vi "GUI.vi"() -> ()   [LabVIEW 2021]
uses:
  <vilib>/Utility/sysdir.llb/System Directory Type.ctl
  Jumps_Globals.vi
  Stevci_Globals.vi
  belezenje.vi
  filePath.vi
  senzorji.vi
  Jump_Globals.vi
  <vilib>/express/express arith-compare/Formula/XNode/ExpressFormulaBlockNode.xnode
panel:
  out "date/time string":string
  out "Time Stamp":timestamp
  out "Start time":string
  in  "?":bool
  out "error out 6":errorcluster
  out "error out 5":errorcluster
  out "error out 4":errorcluster
  out "error out 3":errorcluster
  out "error out 2":errorcluster
  out "error out":errorcluster
  in  "Writing":string[](array[string])
  in  "ID_prejsnji_set6":dbl
  in  "ID_prejsnji_set5":dbl
  in  "ID_prejsnji_set4":dbl
  in  "ID_prejsnji_set3":dbl
  in  "ID_prejsnji_set2":dbl
  in  "ID_prejsnji_set1":dbl
  in  "?":bool
  in  "Lokalni Stevec 6":dbl
  in  "Lokalni Stevec 5":dbl
  in  "Lokalni Stevec 4":dbl
  in  "Lokalni Stevec 3":dbl
  in  "Lokalni Stevec 2":dbl
  in  "?":bool
  in  "Lokalni Stevec":dbl
  in  "?":enum32{"Senzorji", "Tekma", "Set", "Tocka"}(tab)
  out "baterija 6":dbl
  out "baterija 5":dbl
  out "baterija 4":dbl
  out "baterija 3":dbl
  out "baterija 2":dbl
  out "baterija 1":dbl
  out "Senzor 6":bool
  out "Senzor 5":bool
  out "Senzor 4":bool
  out "Senzor 3":bool
  out "Senzor 2":bool
  out "Senzor 1":bool
  out "Stevilo skokov tekma":dbl
  out "Povprecje2_tekma":dbl
  in  "String":string
  out "igralec1":string
  out "igralec2":string
  out "igralec3":string
  out "igralec4":string
  out "igralec5":string
  out "igralec6":string
  in  "String 2":string
  in  "String 3":string
  in  "String 4":string
  in  "String 5":string
  in  "String 6":string
  out "Povprecje1_tekma":dbl
  out "Povprecje3_tekma":dbl
  out "Povprecje4_tekma":dbl
  out "Povprecje5_tekma":dbl
  out "Povprecje6_tekma":dbl
  out "Stevilo skokov tekma 2":dbl
  out "Stevilo skokov tekma 3":dbl
  out "Stevilo skokov tekma 4":dbl
  out "Stevilo skokov tekma 5":dbl
  out "Stevilo skokov tekma 6":dbl
  out "Povprecje2_set":dbl
  out "igralec1 3":string
  out "igralec2 3":string
  out "igralec3 3":string
  out "igralec4 3":string
  out "igralec5 3":string
  out "igralec6 3":string
  in  "String 7":string
  in  "String 18":string
  in  "String 13":string
  in  "String 14":string
  in  "String 11":string
  in  "String 10":string
  out "Povprecje1_set":dbl
  out "Povprecje3_set":dbl
  out "Povprecje4_set":dbl
  out "Povprecje5_set":dbl
  out "Povprecje6_set":dbl
  out "Stevilo skokov set":dbl
  out "Stevilo skokov set 2":dbl
  out "Stevilo skokov set 3":dbl
  out "Stevilo skokov set 4":dbl
  out "Stevilo skokov set 5":dbl
  out "Stevilo skokov set 6":dbl
  out "Povprecje2_tocka":dbl
  out "igralec1 2":string
  out "igralec2 2":string
  out "igralec3 2":string
  out "igralec4 2":string
  out "igralec5 2":string
  out "igralec6 2":string
  in  "String 17":string
  in  "String 16":string
  in  "String 8":string
  in  "String 9":string
  in  "String 15":string
  in  "String 12":string
  out "Povprecje1_tocka":dbl
  out "Povprecje3_tocka":dbl
  out "Povprecje4_tocka":dbl
  out "Povprecje5_tocka":dbl
  out "Povprecje6_tocka":dbl
  out "Stevilo skokov tocka":dbl
  out "Stevilo skokov tocka 2":dbl
  out "Stevilo skokov tocka 3":dbl
  out "Stevilo skokov tocka 4":dbl
  out "Stevilo skokov tocka 5":dbl
  out "Stevilo skokov tocka 6":dbl
  out "path":path
  # "SENZORJE JE POTREBNO PRED PONOVNIM ZACETKOM  UGASNITI IN PONOVNO PRIŽGATI DA SE POMNILNIK IZBRIŠE"
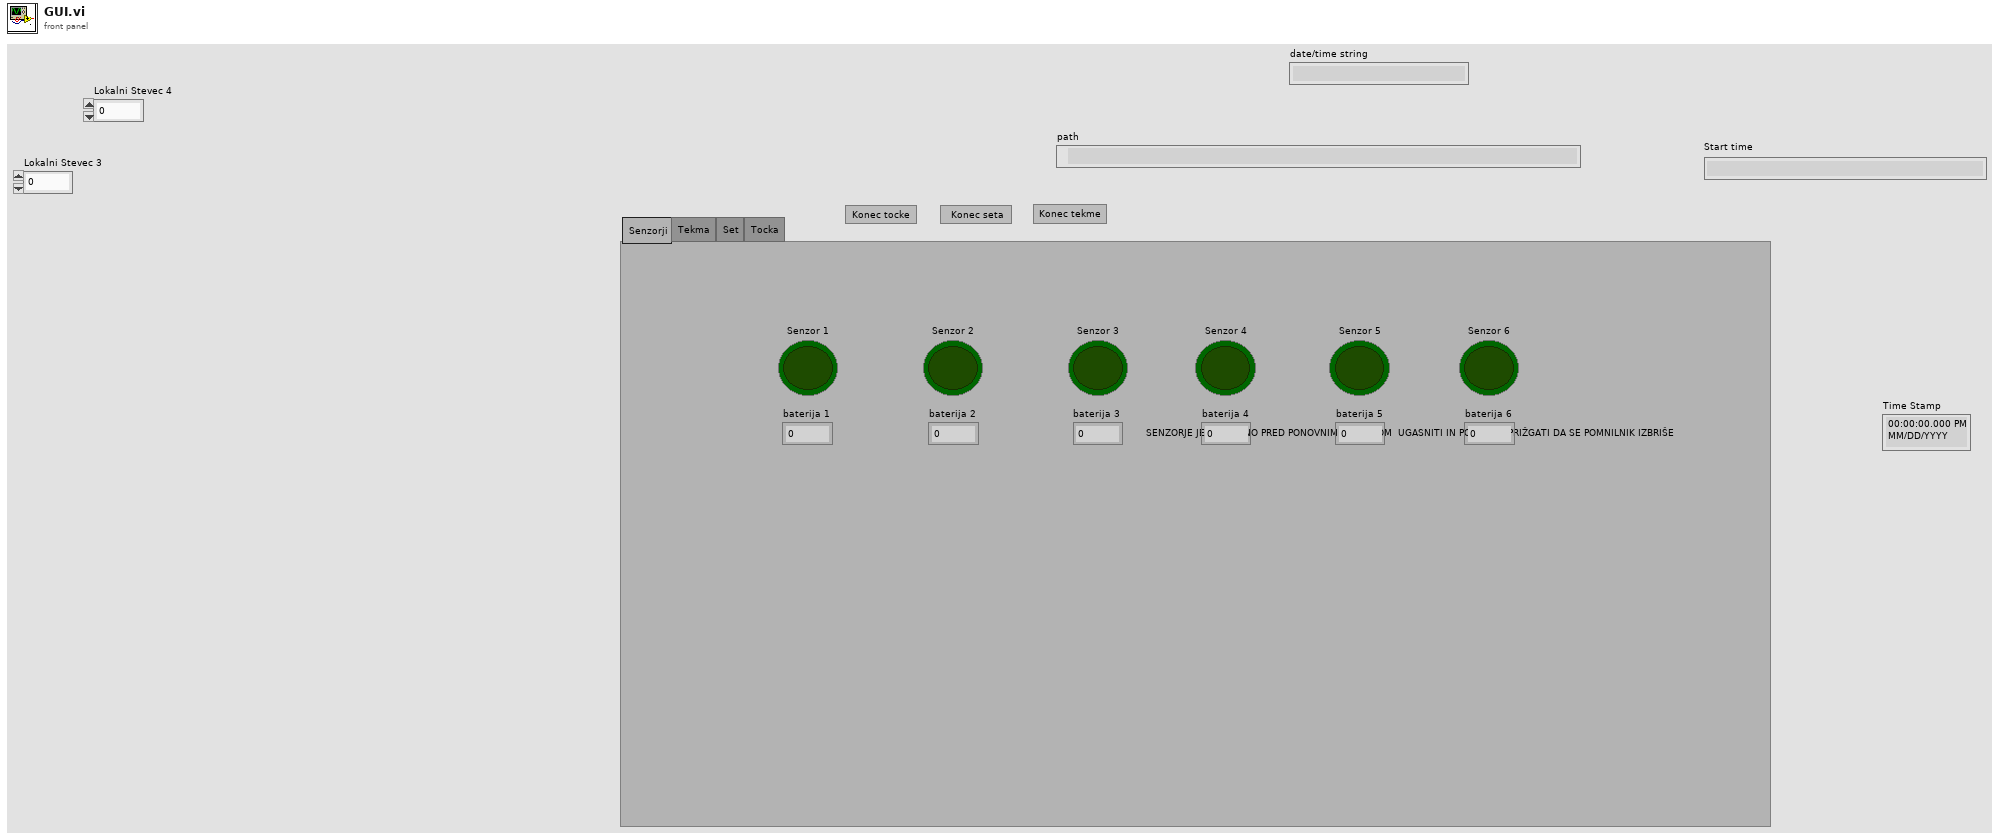
[diagram p1: front panel]
types:
  T1 = typedef "System Directory Type.ctl" = i32
  T2 = enum16{"open", "open or create", "create or replace", "create", "open (read-only)"}
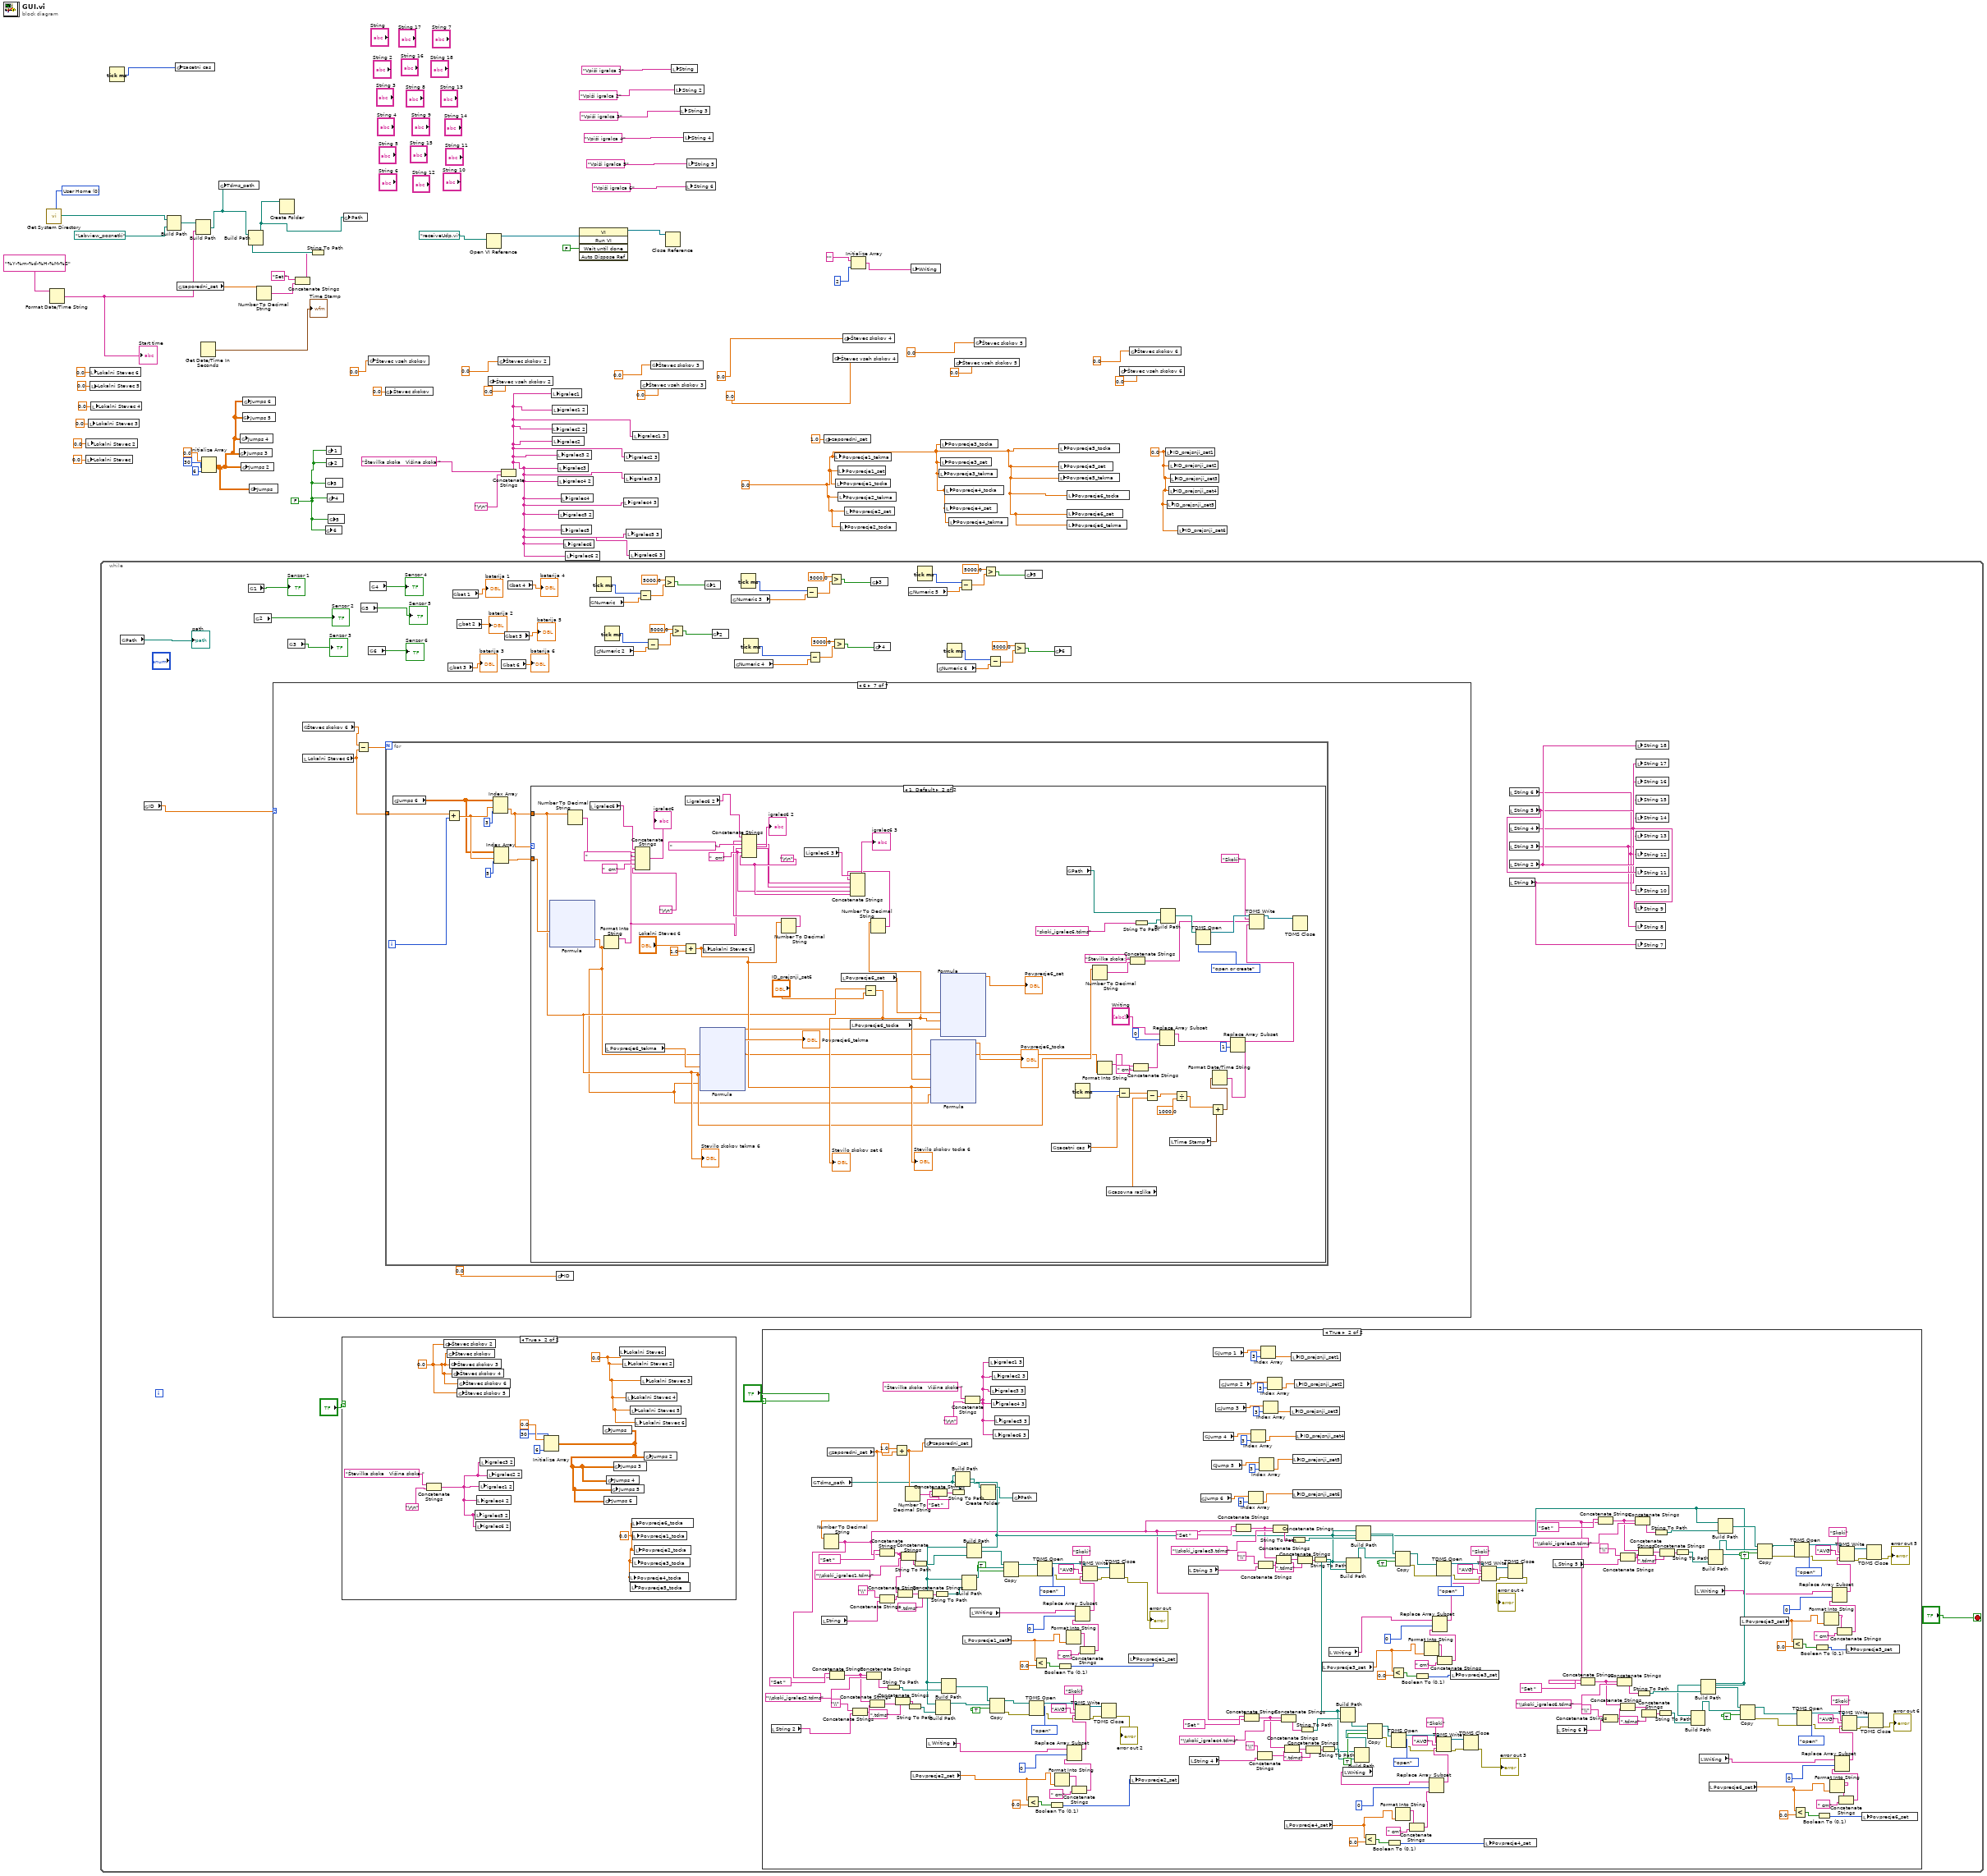
[diagram p0: block diagram]
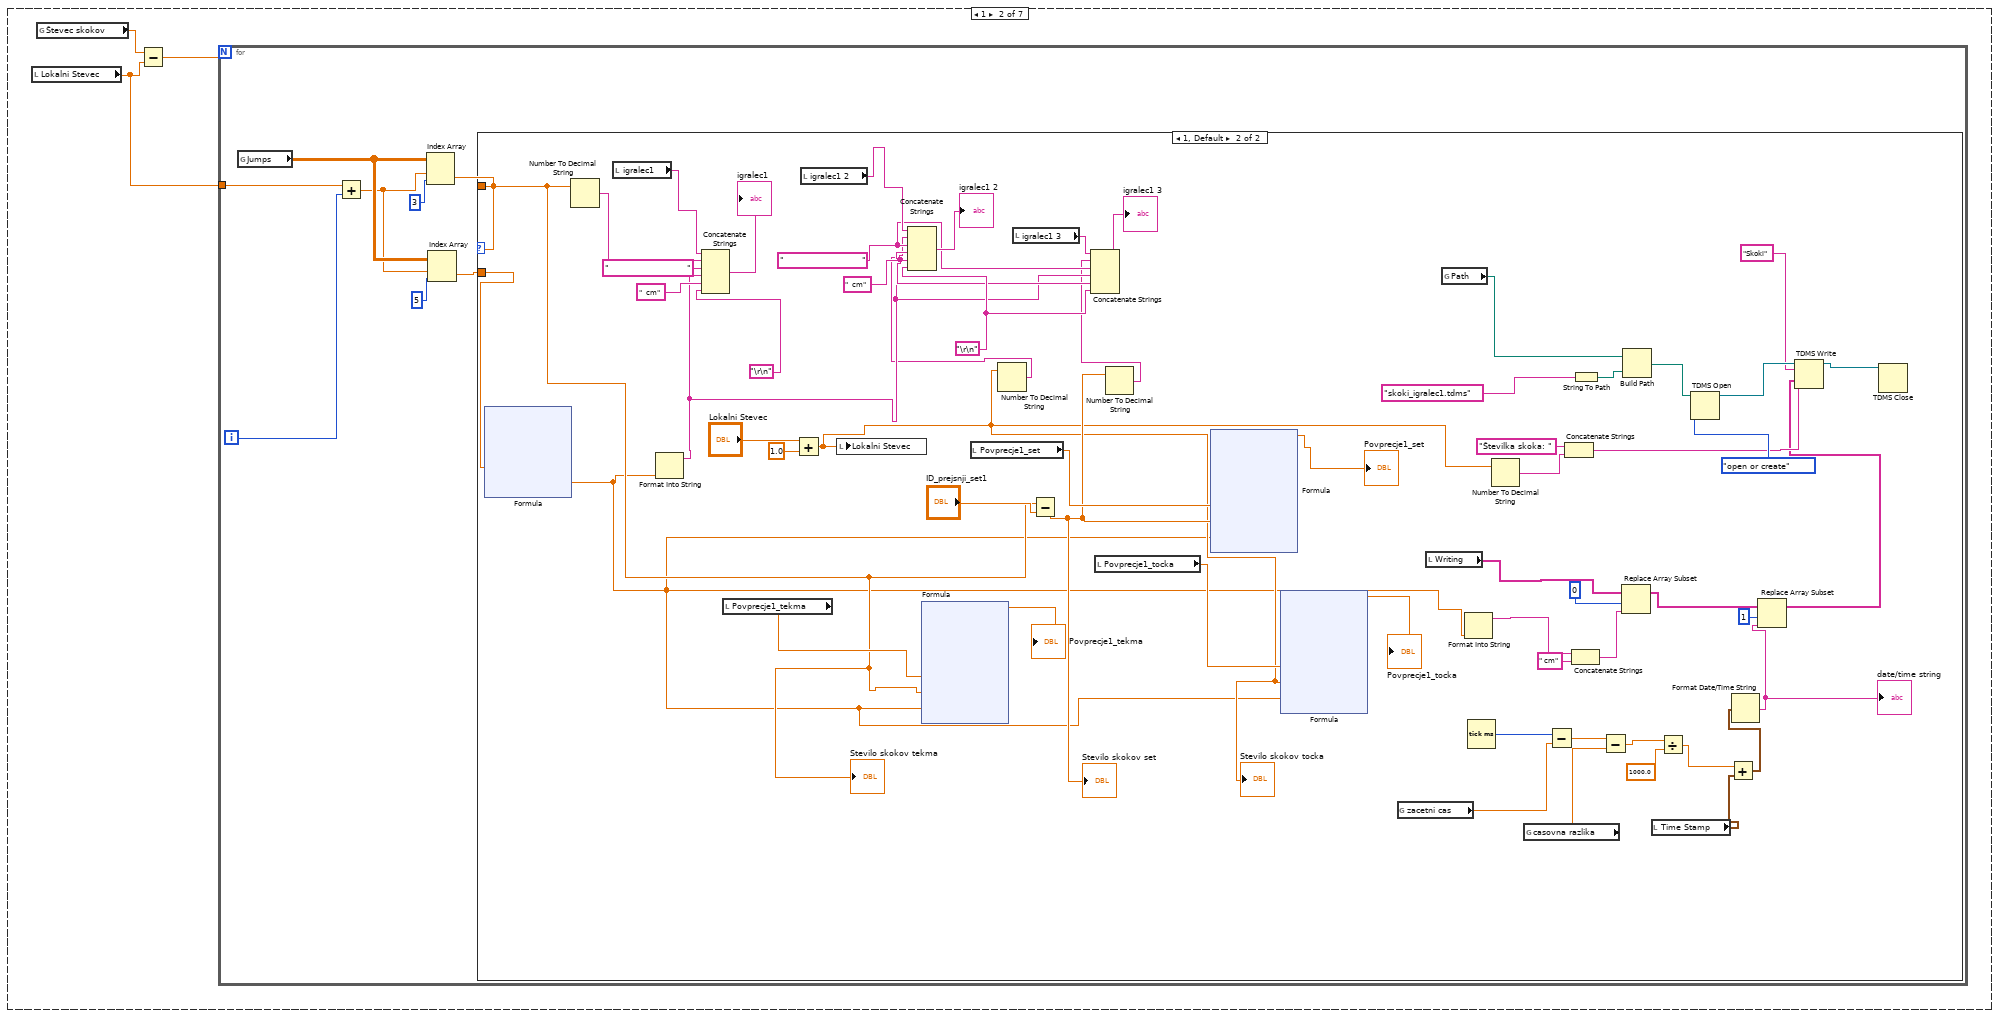
[diagram p5: hidden frame]
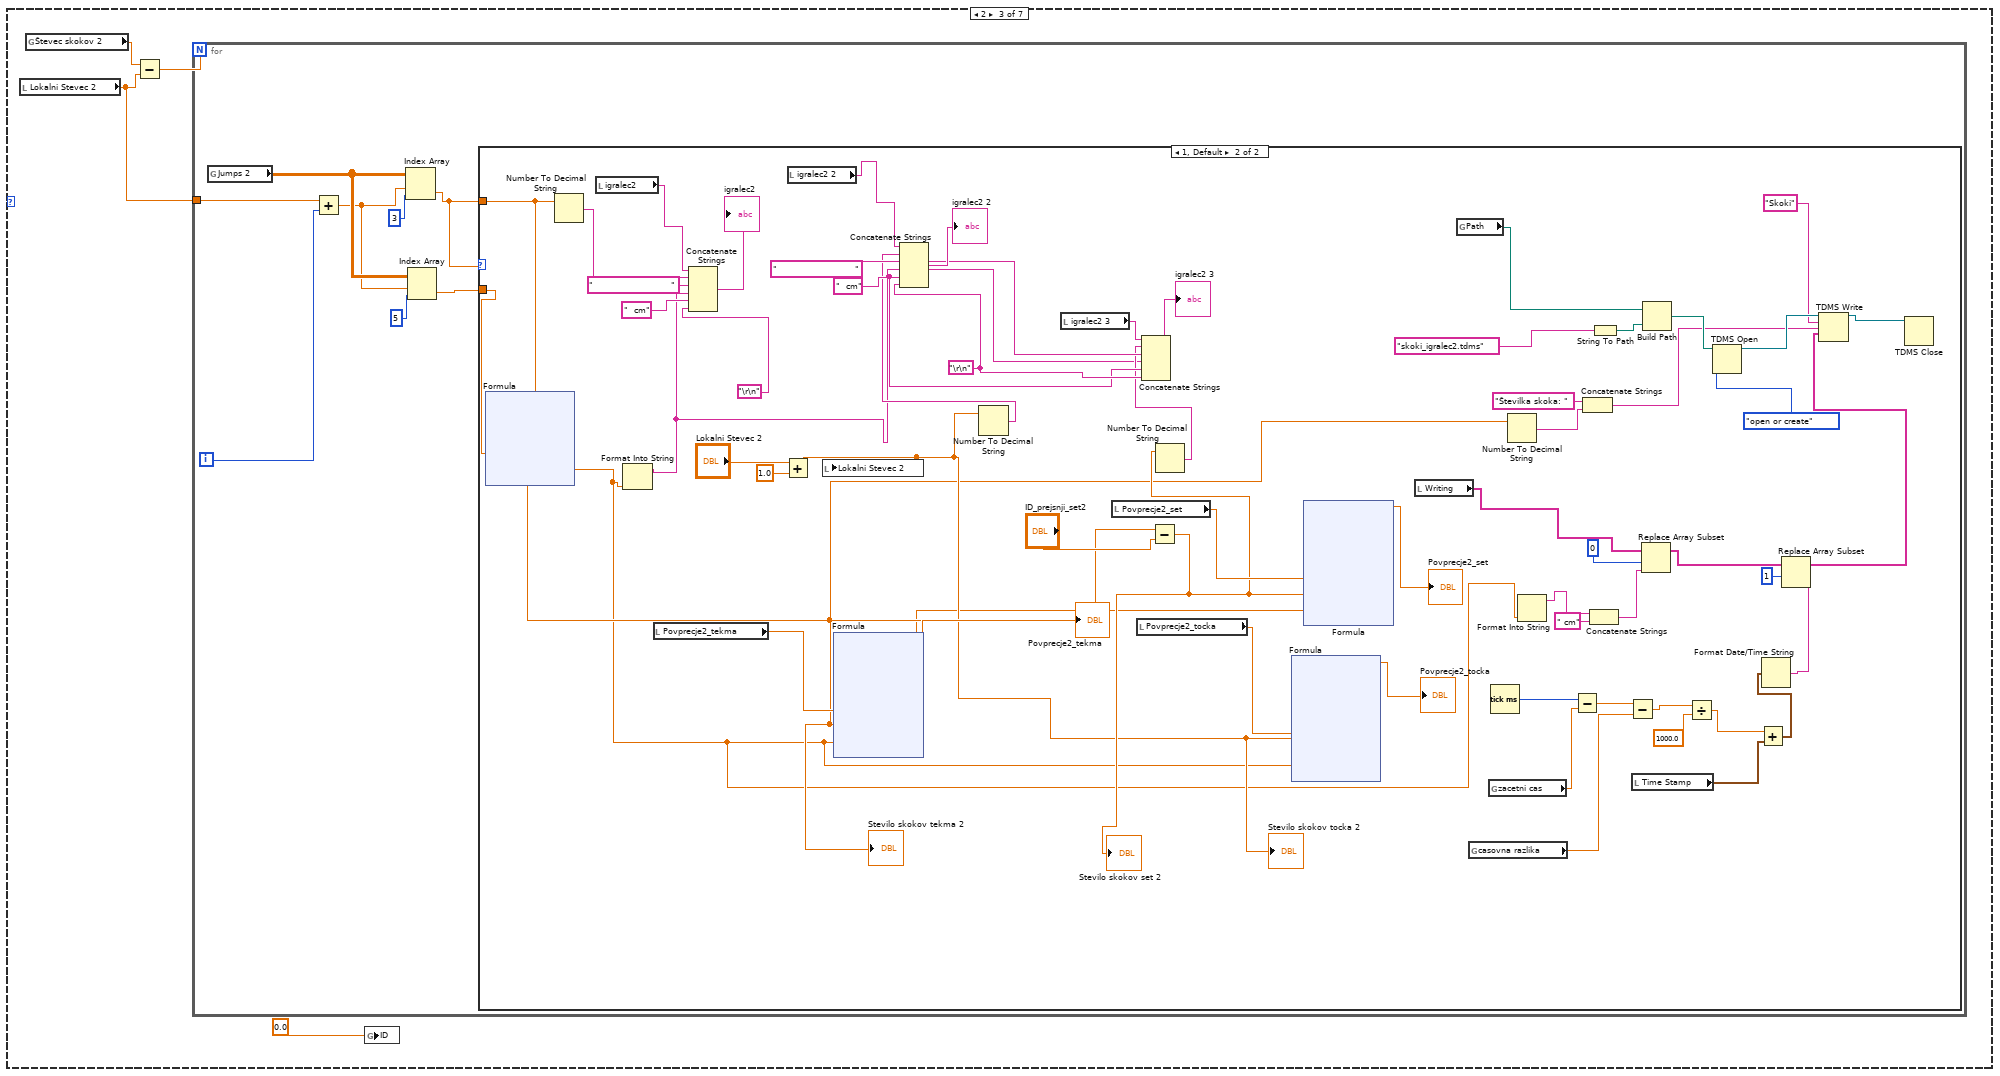
[diagram p7: hidden frame]
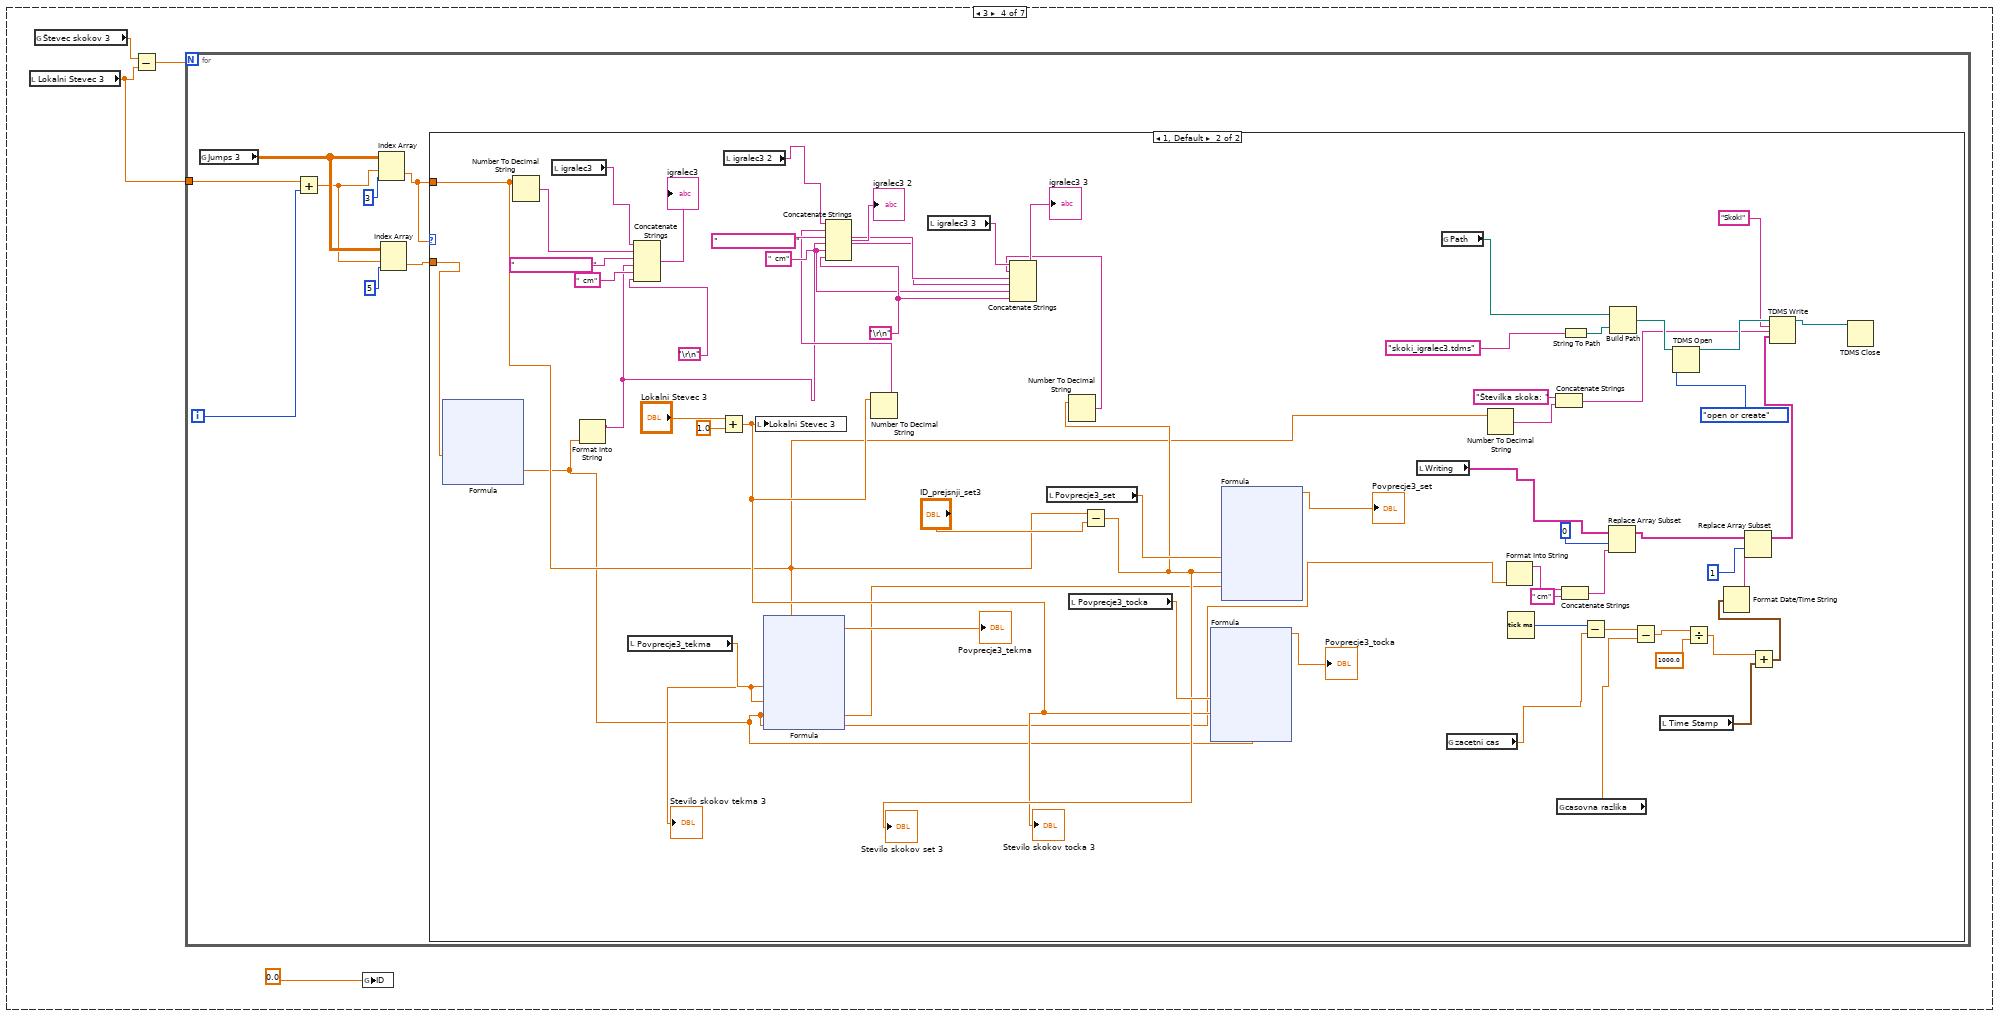
[diagram p9: hidden frame]
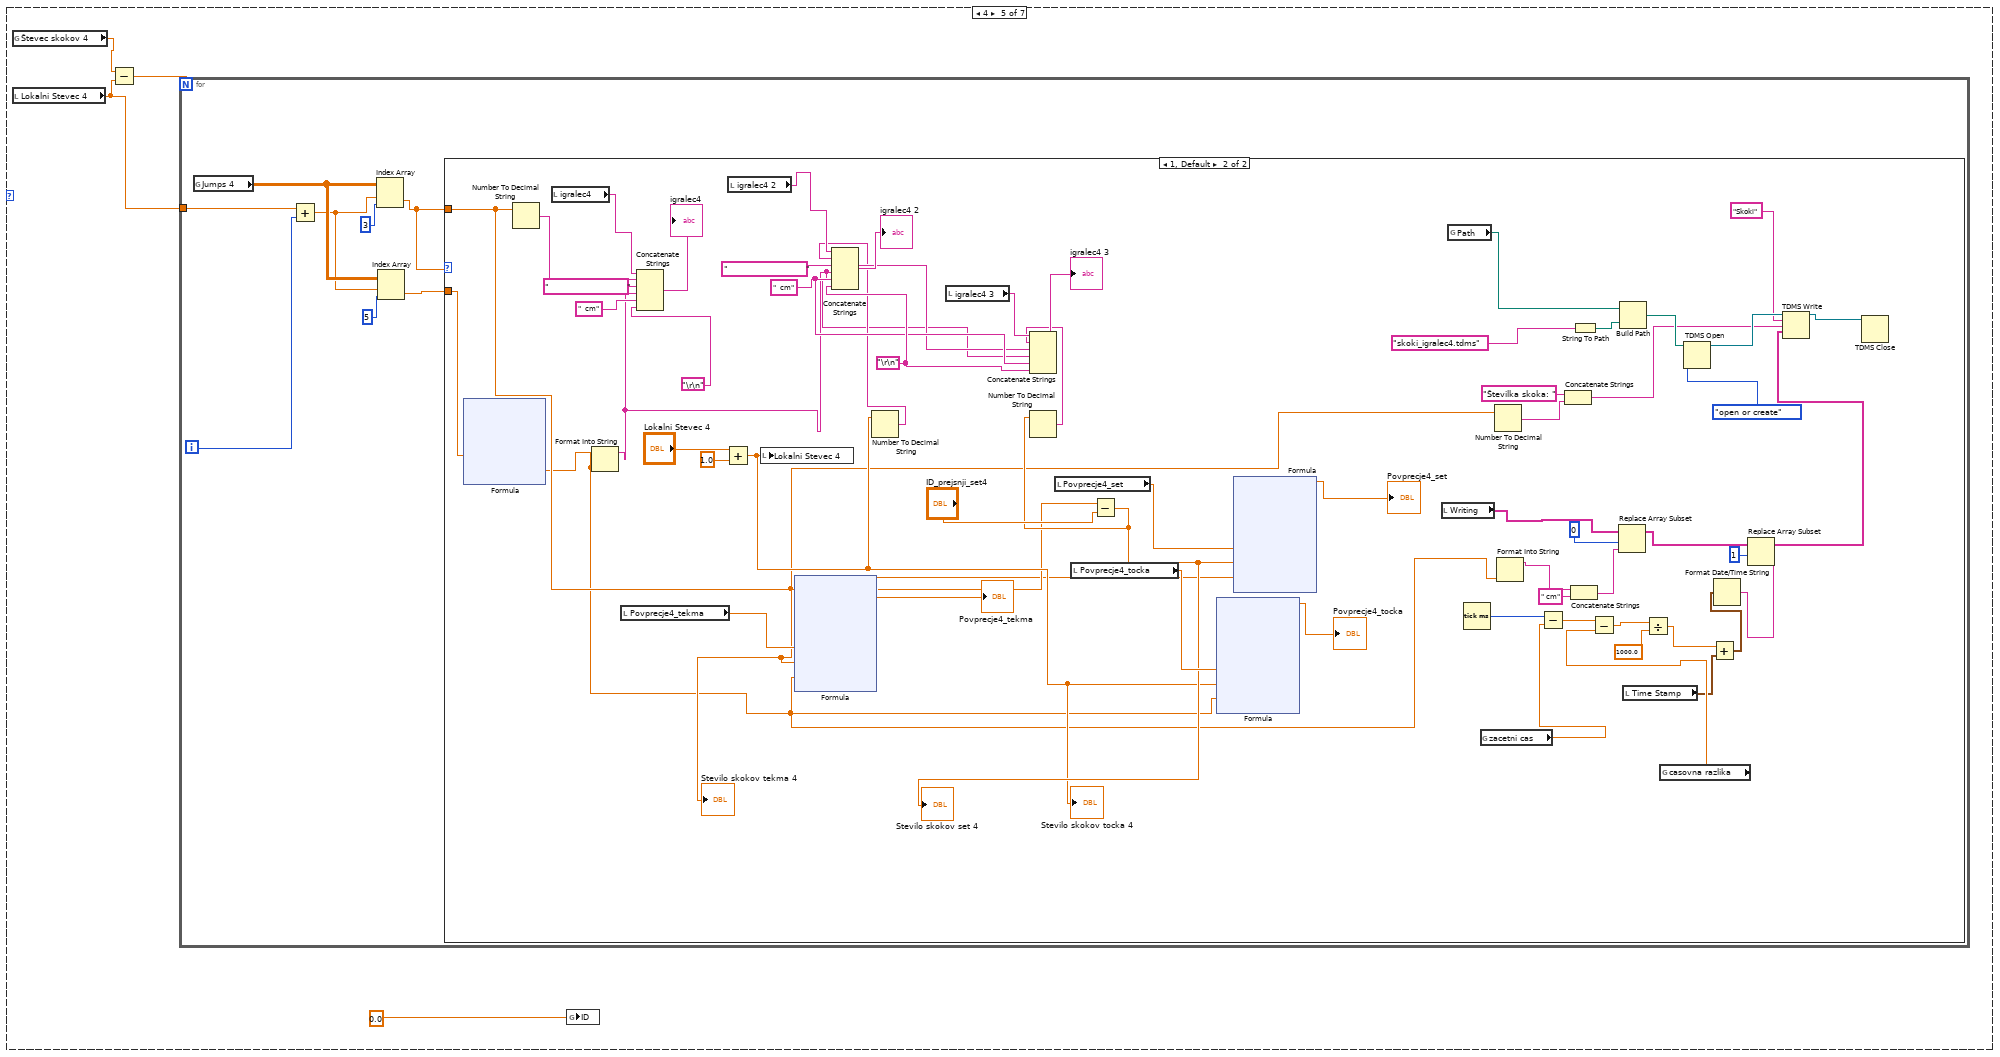
[diagram p11: hidden frame]
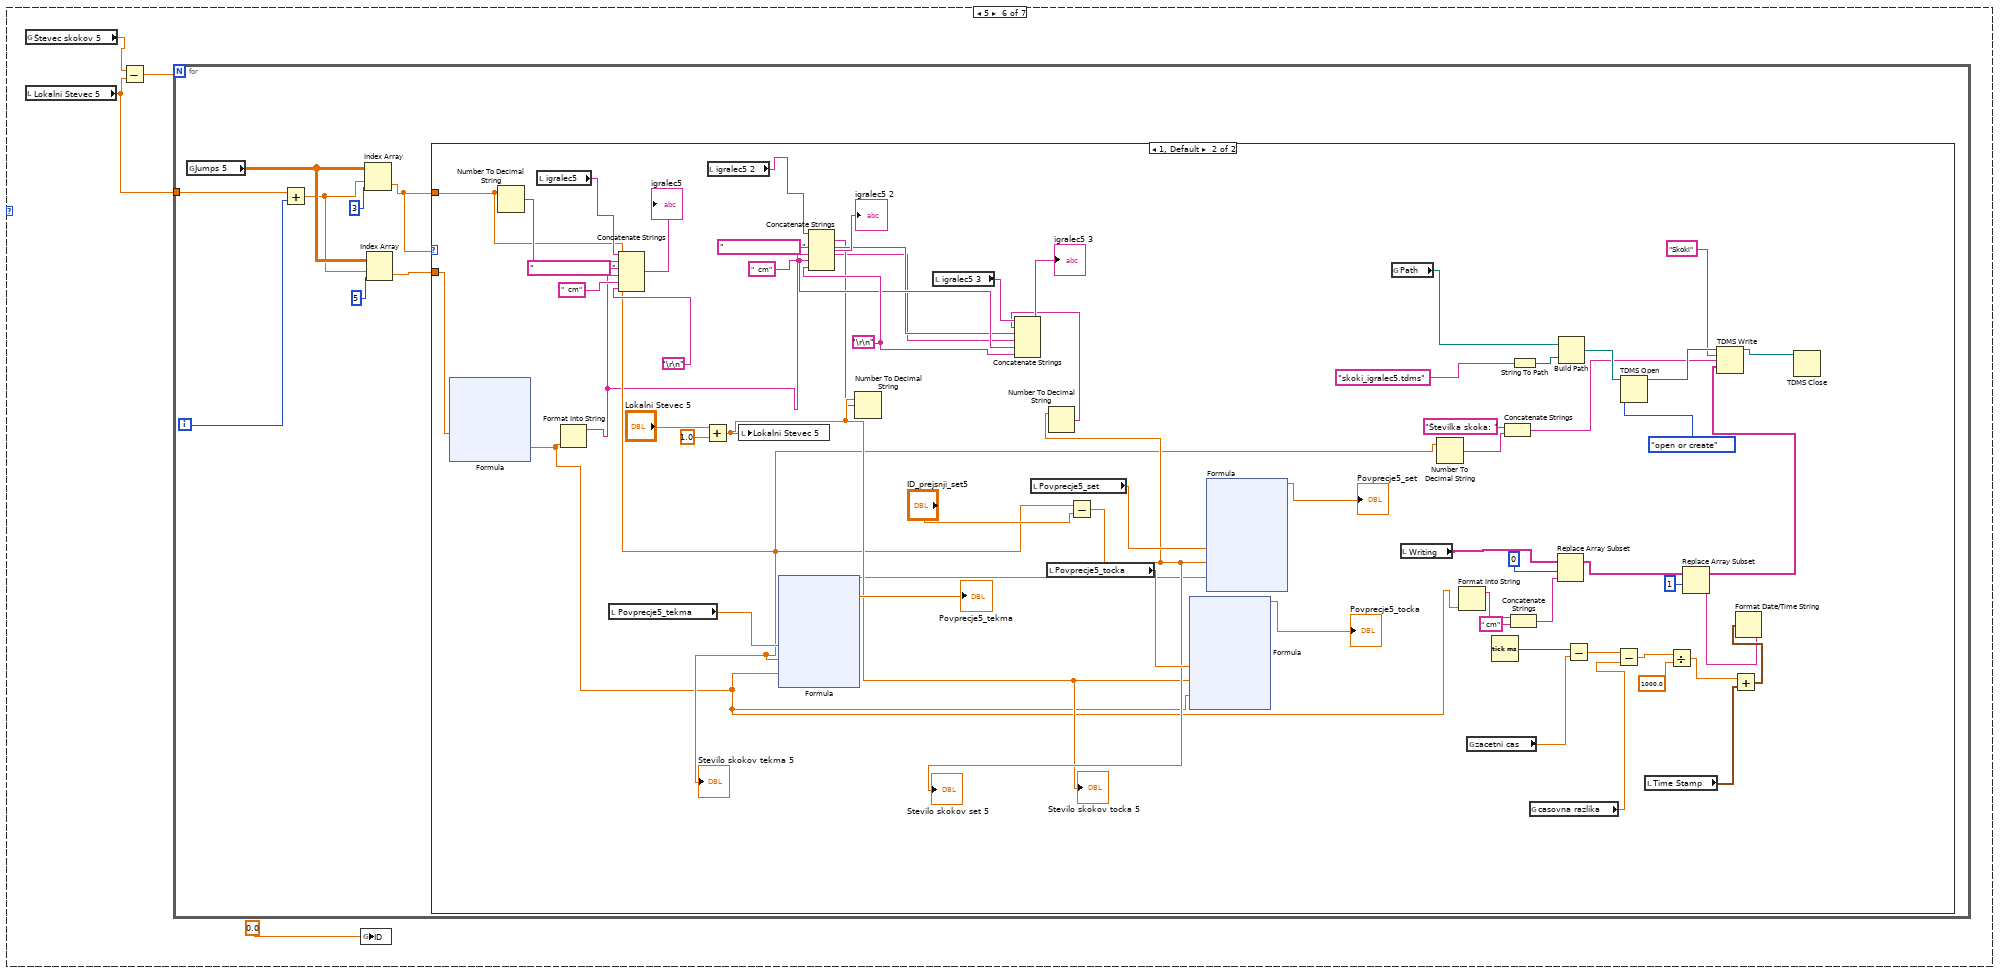
[diagram p13: hidden frame]
diagram:
  w3 = FALSE ("Senzor 6")
  w8 = 0.0 ("ID_prejsnji_set1")
  w9 = 0.0 ("Povprecje_1_tocka")
  w27 = T1 0 items=["User Home"=0, "User Desktop"=1, "User Documents"=2, "User Application Data"=3, "User Preferences"=4, "User Temporary"=5, "Public Documents"=6, "Public Application Data"=7, "Public Preferences"=8, "Public Cache"=13, "System Core Libraries"=9, "System Installed Libraries"=10, "Application Files"=11, "Boot Volume Root"=12] ("system directory type")
  n1 = call <vilib>:"Get System Directory.vi"("system directory type"=w27) -> ("system directory"=w26:path)  [unwired: 10 in]
  n2 = Format Date/Time String(time format string (%c)="%Y-%m-%d-%H-%M-%S") -> (date/time string=w2:string)  [unwired: 2 in]
  "Start time" <- w2
  n3 = local write "Lokalni Stevec"(0.0 ("Lokalni Stevec")) -> ()
  n4 = local write "Lokalni Stevec 2"(0.0 ("Lokalni Stevec 2")) -> ()
  n5 = local write "Lokalni Stevec 3"(0.0 ("Lokalni Stevec 3")) -> ()
  n6 = local write "Lokalni Stevec 6"(0.0 ("Lokalni Stevec 6")) -> ()
  n7 = local write "Lokalni Stevec 5"(0.0 ("Lokalni Stevec 5")) -> ()
  n8 = local write "Lokalni Stevec 4"(0.0 ("Lokalni Stevec 4")) -> ()
  n9 = while {
    stop <- "?" stop-if-true
    n10 = global read "filePath.vi" "Path"() -> (→"path":path)
    n11 = global read "belezenje.vi" "ID"() -> (w108:dbl)
    n12 = global read "senzorji.vi" "1"() -> (→"Senzor 1":bool)
    n13 = global read "senzorji.vi" "2"() -> (→"Senzor 2":bool)
    n14 = case shown="6" w108 {
      frame 0, Default {
      }
      frame 1 {
        n15 = local read "Lokalni Stevec"() -> (w363:dbl)
        n16 = global read "Stevci_Globals.vi" "Števec skokov"() -> (w365:dbl)
        n17 = Subtract(x=w365, y=w363) -> (x-y=w364:dbl)
        n18 = for {
          N: w364 -> [_]
          tunnel: w363 -> [w372]
          i -> [w367]
          n19 = global read "Jumps_Globals.vi" "Jumps"() -> (w370:dbl[][])
          n20 = Add(x=w372, y=w367) -> (x+y=w369:dbl)
          n21 = Index Array(array=w370, index (row)=w369, index (col)=3 ("index")) -> (element=w366:dbl)
          n22 = Index Array(array=w370, index (row)=w369, index (col)=5 ("index")) -> (element=w368:dbl)
          n23 = case shown="1, Default" w366 {
            tunnel: w366 -> [_ w382]
            tunnel: w368 -> [_ w429]
            frame 0 {
            }
            frame 1, Default {
              w421 = "  cm" ("string")
              w420 = "                          " ("string")
              w422 = "\r\n"
              n24 = xnode "Formula"("X1"=w429) -> ("Result"=w381:dbl)  [unwired: 1 in, 1 out]
              n25 = Number To Decimal String(number=w382) -> (decimal integer string=w419:string)  [unwired: 1 in]
              n26 = local read "igralec1"() -> (w432:string)
              n27 = Format Into String(w381) -> (resulting string=w416:string)  [unwired: 3 in, 1 out]
              n28 = Concatenate Strings(w432, w419, "                          " ("string"), w416, "  cm" ("string"), "\r\n") -> (→"igralec1":string)
              n29 = local read "Povprecje1_tekma"() -> (w415:dbl)
              n30 = Add(x="Lokalni Stevec", y=1.0) -> (x+y=w383:dbl)
              "Stevilo skokov tocka" <- w383
              n31 = local read "igralec1 2"() -> (w423:string)
              n32 = local write "Lokalni Stevec"(w383) -> ()
              n33 = xnode "Formula"("X1"=w415, "X2"=w382, "X3"=w381) -> ("Result"=→"Povprecje1_tekma":dbl)  [unwired: 1 in, 1 out]
              n34 = local read "Povprecje1_set"() -> (w412:dbl)
              n35 = Number To Decimal String(number=w383) -> (decimal integer string=w406:string)  [unwired: 1 in]
              n36 = Concatenate Strings(w423, w406, w420, w416, w421, w422) -> (→"igralec1 2":string)
              n37 = local read "igralec1 3"() -> (w417:string)
              n38 = Subtract(x=w382, y="ID_prejsnji_set1") -> (x-y=w408:dbl)
              "Stevilo skokov set" <- w408
              n39 = local read "Povprecje1_tocka"() -> (w410:dbl)
              n40 = Number To Decimal String(number=w408) -> (decimal integer string=w407:string)  [unwired: 1 in]
              n41 = Concatenate Strings(w417, w407, w420, w416, w421, w422) -> (→"igralec1 3":string)
              n42 = xnode "Formula"("X1"=w412, "X2"=w408, "X3"=w381) -> ("Result"=→"Povprecje1_set":dbl)  [unwired: 1 in, 1 out]
              n43 = xnode "Formula"("X1"=w410, "X2"=w383, "X3"=w381) -> ("Result"=→"Povprecje1_tocka":dbl)  [unwired: 1 in, 1 out]
              n44 = global read "Stevci_Globals.vi" "zacetni cas"() -> (w389:dbl)
              n45 = local read "Writing"() -> (w384:string[])
              n46 = global read "filePath.vi" "Path"() -> (w401:path)
              n47 = Format Into String(w381) -> (resulting string=w380:string)  [unwired: 3 in, 1 out]
              n48 = Tick Count (ms)() -> (millisecond timer value=w388:u32)
              n49 = Number To Decimal String(number=w383) -> (decimal integer string=w398:string)  [unwired: 1 in]
              n50 = global read "Stevci_Globals.vi" "casovna razlika"() -> (w387:dbl)
              n51 = Subtract(x=w388, y=w389) -> (x-y=w386:dbl)
              n52 = Concatenate Strings("Številka skoka: " ("string"), w398) -> (w395:string)
              n53 = Concatenate Strings(w380, " cm" ("string")) -> (w394:string)
              n54 = String To Path(string="skoki_igralec1.tdms") -> (path=w403:path)
              n55 = Subtract(x=w386, y=w387) -> (x-y=w379:dbl)
              n56 = Replace Array Subset(array=w384, new element=w394, index=0) -> (w392:string[])
              n57 = Build Path(base path=w401, name or relative path=w403) -> (appended path=w404:path)
              n58 = local read "Time Stamp"() -> (w376:timestamp)
              n59 = Divide(x=w379, y=1000.0) -> (x/y=w377:dbl)
              n60 = TDMS Open(10:T2."open or create" ("operation (0:open)"), 11:w404) -> (3:w405:refnum<k34>)  [unwired: 5 in, 1 out]
              n61 = Add(x=w377, y=w376) -> (x+y=w375:timestamp)
              n62 = Format Date/Time String(seconds (now)=w375) -> (date/time string=w374:string)  [unwired: 2 in]
              "date/time string" <- w374
              n63 = Replace Array Subset(array=w392, new element=w374, index=1) -> (w390:string[])
              n64 = TDMS Write(0:w405, 5:"Skoki" ("group name in (Untitled)"), 7:w395, 9:w390) -> (4:w385:refnum<k34>)  [unwired: 2 in, 3 out]
              n65 = TDMS Close(11:w385) -> ()  [unwired: 1 in, 2 out]
              "Stevilo skokov tekma" <- w382
            }
          }
        }
      }
      frame 2 {
        n66 = local read "Lokalni Stevec 2"() -> (w478:dbl)
        n67 = global read "Stevci_Globals.vi" "Števec skokov 2"() -> (w480:dbl)
        n68 = Subtract(x=w480, y=w478) -> (x-y=w479:dbl)
        n69 = for {
          N: w479 -> [_]
          tunnel: w478 -> [w485]
          i -> [w486]
          n70 = global read "Jumps_Globals.vi" "Jumps 2"() -> (w483:dbl[][])
          n71 = Add(x=w485, y=w486) -> (x+y=w482:dbl)
          n72 = Index Array(array=w483, index (row)=w482, index (col)=3 ("index")) -> (element=w488:dbl)
          n73 = Index Array(array=w483, index (row)=w482, index (col)=5 ("index")) -> (element=w481:dbl)
          n74 = case shown="1, Default" w488 {
            tunnel: w488 -> [_ w503]
            tunnel: w481 -> [_ w544]
            frame 0 {
            }
            frame 1, Default {
              w534 = "  cm" ("string")
              w533 = "                          " ("string")
              w535 = "\r\n"
              n75 = xnode "Formula"("X1"=w544) -> ("Result"=w500:dbl)  [unwired: 1 in, 1 out]
              n76 = Number To Decimal String(number=w503) -> (decimal integer string=w532:string)  [unwired: 1 in]
              n77 = local read "igralec2"() -> (w547:string)
              n78 = Format Into String(w500) -> (resulting string=w501:string)  [unwired: 3 in, 1 out]
              n79 = local read "Povprecje2_tekma"() -> (w530:dbl)
              n80 = Concatenate Strings(w547, w532, "                          " ("string"), w501, "  cm" ("string"), "\r\n") -> (→"igralec2":string)
              n81 = Add(x="Lokalni Stevec 2", y=1.0) -> (x+y=w522:dbl)
              "Stevilo skokov tocka 2" <- w522
              n82 = local read "igralec2 2"() -> (w538:string)
              n83 = local write "Lokalni Stevec 2"(w522) -> ()
              n84 = xnode "Formula"("X1"=w530, "X2"=w503, "X3"=w500) -> ("Result"=→"Povprecje2_tekma":dbl)  [unwired: 1 in, 1 out]
              n85 = Number To Decimal String(number=w522) -> (decimal integer string=w521:string)  [unwired: 1 in]
              n86 = Concatenate Strings(w538, w521, w533, w501, w534, w535) -> (→"igralec2 2":string)
              n87 = local read "igralec2 3"() -> (w536:string)
              n88 = local read "Povprecje2_set"() -> (w528:dbl)
              n89 = local read "Povprecje2_tocka"() -> (w527:dbl)
              n90 = Subtract(x=w503, y="ID_prejsnji_set2") -> (x-y=w524:dbl)
              "Stevilo skokov set 2" <- w524
              n91 = Number To Decimal String(number=w524) -> (decimal integer string=w523:string)  [unwired: 1 in]
              n92 = Concatenate Strings(w536, w523, w533, w501, w534, w535) -> (→"igralec2 3":string)
              n93 = xnode "Formula"("X1"=w527, "X2"=w522, "X3"=w500) -> ("Result"=→"Povprecje2_tocka":dbl)  [unwired: 1 in, 1 out]
              n94 = xnode "Formula"("X1"=w528, "X2"=w524, "X3"=w500) -> ("Result"=→"Povprecje2_set":dbl)  [unwired: 1 in, 1 out]
              n95 = local read "Writing"() -> (w502:string[])
              n96 = global read "filePath.vi" "Path"() -> (w516:path)
              n97 = global read "Stevci_Globals.vi" "casovna razlika"() -> (w492:dbl)
              n98 = global read "Stevci_Globals.vi" "zacetni cas"() -> (w491:dbl)
              n99 = Tick Count (ms)() -> (millisecond timer value=w498:u32)
              n100 = Number To Decimal String(number=w503) -> (decimal integer string=w513:string)  [unwired: 1 in]
              n101 = Format Into String(w500) -> (resulting string=w499:string)  [unwired: 3 in, 1 out]
              n102 = Subtract(x=w498, y=w491) -> (x-y=w497:dbl)
              n103 = Concatenate Strings("Številka skoka: " ("string"), w513) -> (w510:string)
              n104 = Concatenate Strings(w499, " cm" ("string")) -> (w509:string)
              n105 = String To Path(string="skoki_igralec2.tdms") -> (path=w518:path)
              n106 = Subtract(x=w497, y=w492) -> (x-y=w496:dbl)
              n107 = local read "Time Stamp"() -> (w490:timestamp)
              n108 = Replace Array Subset(array=w502, new element=w509, index=0) -> (w507:string[])
              n109 = Build Path(base path=w516, name or relative path=w518) -> (appended path=w519:path)
              n110 = Divide(x=w496, y=1000.0) -> (x/y=w494:dbl)
              n111 = TDMS Open(10:T2."open or create" ("operation (0:open)"), 11:w519) -> (3:w520:refnum<k34>)  [unwired: 5 in, 1 out]
              n112 = Add(x=w494, y=w490) -> (x+y=w493:timestamp)
              n113 = Format Date/Time String(seconds (now)=w493) -> (date/time string=w489:string)  [unwired: 2 in]
              n114 = Replace Array Subset(array=w507, new element=w489, index=1) -> (w505:string[])
              n115 = TDMS Write(0:w520, 5:"Skoki" ("group name in (Untitled)"), 7:w510, 9:w505) -> (4:w504:refnum<k34>)  [unwired: 2 in, 3 out]
              n116 = TDMS Close(11:w504) -> ()  [unwired: 1 in, 2 out]
              "Stevilo skokov tekma 2" <- w503
            }
          }
        }
        n117 = global write "belezenje.vi" "ID"(0.0 ("ID")) -> ()
      }
      frame 3 {
        n118 = local read "Lokalni Stevec 3"() -> (w593:dbl)
        n119 = global read "Stevci_Globals.vi" "Števec skokov 3"() -> (w595:dbl)
        n120 = Subtract(x=w595, y=w593) -> (x-y=w594:dbl)
        n121 = for {
          N: w594 -> [_]
          tunnel: w593 -> [w600]
          i -> [w601]
          n122 = global read "Jumps_Globals.vi" "Jumps 3"() -> (w598:dbl[][])
          n123 = Add(x=w600, y=w601) -> (x+y=w597:dbl)
          n124 = Index Array(array=w598, index (row)=w597, index (col)=3 ("index")) -> (element=w603:dbl)
          n125 = Index Array(array=w598, index (row)=w597, index (col)=5 ("index")) -> (element=w596:dbl)
          n126 = case shown="1, Default" w603 {
            tunnel: w603 -> [_ w619]
            tunnel: w596 -> [_ w659]
            frame 0 {
            }
            frame 1, Default {
              w649 = "  cm" ("string")
              w648 = "                          " ("string")
              w650 = "\r\n"
              n127 = xnode "Formula"("X1"=w659) -> ("Result"=w615:dbl)  [unwired: 1 in, 1 out]
              n128 = Number To Decimal String(number=w619) -> (decimal integer string=w647:string)  [unwired: 1 in]
              n129 = local read "igralec3"() -> (w662:string)
              n130 = Format Into String(w615) -> (resulting string=w616:string)  [unwired: 3 in, 1 out]
              n131 = local read "Povprecje3_tekma"() -> (w645:dbl)
              n132 = Concatenate Strings(w662, w647, "                          " ("string"), w616, "  cm" ("string"), "\r\n") -> (→"igralec3":string)
              n133 = Add(x="Lokalni Stevec 3", y=1.0) -> (x+y=w637:dbl)
              "Stevilo skokov tocka 3" <- w637
              n134 = local read "igralec3 2"() -> (w653:string)
              n135 = local write "Lokalni Stevec 3"(w637) -> ()
              n136 = xnode "Formula"("X1"=w645, "X2"=w619, "X3"=w615) -> ("Result"=→"Povprecje3_tekma":dbl)  [unwired: 1 in, 1 out]
              n137 = Number To Decimal String(number=w637) -> (decimal integer string=w636:string)  [unwired: 1 in]
              n138 = Concatenate Strings(w653, w636, w648, w616, w649, w650) -> (→"igralec3 2":string)
              n139 = local read "igralec3 3"() -> (w651:string)
              n140 = local read "Povprecje3_set"() -> (w644:dbl)
              n141 = local read "Povprecje3_tocka"() -> (w643:dbl)
              n142 = Subtract(x=w619, y="ID_prejsnji_set3") -> (x-y=w639:dbl)
              "Stevilo skokov set 3" <- w639
              n143 = Number To Decimal String(number=w639) -> (decimal integer string=w638:string)  [unwired: 1 in]
              n144 = Concatenate Strings(w651, w638, w648, w616, w649, w650) -> (→"igralec3 3":string)
              n145 = xnode "Formula"("X1"=w643, "X2"=w637, "X3"=w615) -> ("Result"=→"Povprecje3_tocka":dbl)  [unwired: 1 in, 1 out]
              n146 = xnode "Formula"("X1"=w644, "X2"=w639, "X3"=w615) -> ("Result"=→"Povprecje3_set":dbl)  [unwired: 1 in, 1 out]
              n147 = local read "Writing"() -> (w617:string[])
              n148 = global read "filePath.vi" "Path"() -> (w631:path)
              n149 = global read "Stevci_Globals.vi" "zacetni cas"() -> (w607:dbl)
              n150 = Number To Decimal String(number=w619) -> (decimal integer string=w628:string)  [unwired: 1 in]
              n151 = Format Into String(w615) -> (resulting string=w614:string)  [unwired: 3 in, 1 out]
              n152 = Tick Count (ms)() -> (millisecond timer value=w613:u32)
              n153 = Concatenate Strings("Številka skoka: " ("string"), w628) -> (w625:string)
              n154 = global read "Stevci_Globals.vi" "casovna razlika"() -> (w606:dbl)
              n155 = Concatenate Strings(w614, " cm" ("string")) -> (w624:string)
              n156 = String To Path(string="skoki_igralec3.tdms") -> (path=w633:path)
              n157 = Subtract(x=w613, y=w607) -> (x-y=w612:dbl)
              n158 = Replace Array Subset(array=w617, new element=w624, index=0) -> (w618:string[])
              n159 = Build Path(base path=w631, name or relative path=w633) -> (appended path=w634:path)
              n160 = Subtract(x=w612, y=w606) -> (x-y=w611:dbl)
              n161 = local read "Time Stamp"() -> (w605:timestamp)
              n162 = TDMS Open(10:T2."open or create" ("operation (0:open)"), 11:w634) -> (3:w635:refnum<k34>)  [unwired: 5 in, 1 out]
              n163 = Divide(x=w611, y=1000.0) -> (x/y=w609:dbl)
              n164 = Add(x=w609, y=w605) -> (x+y=w608:timestamp)
              n165 = Format Date/Time String(seconds (now)=w608) -> (date/time string=w604:string)  [unwired: 2 in]
              n166 = Replace Array Subset(array=w618, new element=w604, index=1) -> (w621:string[])
              n167 = TDMS Write(0:w635, 5:"Skoki" ("group name in (Untitled)"), 7:w625, 9:w621) -> (4:w620:refnum<k34>)  [unwired: 2 in, 3 out]
              n168 = TDMS Close(11:w620) -> ()  [unwired: 1 in, 2 out]
              "Stevilo skokov tekma 3" <- w619
            }
          }
        }
        n169 = global write "belezenje.vi" "ID"(0.0 ("ID")) -> ()
      }
      frame 4 {
        n170 = global read "Stevci_Globals.vi" "Števec skokov 4"() -> (w710:dbl)
        n171 = local read "Lokalni Stevec 4"() -> (w708:dbl)
        n172 = Subtract(x=w710, y=w708) -> (x-y=w709:dbl)
        n173 = for {
          N: w709 -> [_]
          tunnel: w708 -> [w715]
          i -> [w716]
          n174 = global read "Jumps_Globals.vi" "Jumps 4"() -> (w713:dbl[][])
          n175 = Add(x=w715, y=w716) -> (x+y=w712:dbl)
          n176 = Index Array(array=w713, index (row)=w712, index (col)=3 ("index")) -> (element=w718:dbl)
          n177 = Index Array(array=w713, index (row)=w712, index (col)=5 ("index")) -> (element=w711:dbl)
          n178 = case shown="1, Default" w718 {
            tunnel: w718 -> [_ w733]
            tunnel: w711 -> [_ w774]
            frame 0 {
            }
            frame 1, Default {
              w764 = "  cm" ("string")
              w763 = "                          " ("string")
              w765 = "\r\n"
              n179 = xnode "Formula"("X1"=w774) -> ("Result"=w730:dbl)  [unwired: 1 in, 1 out]
              n180 = Number To Decimal String(number=w733) -> (decimal integer string=w762:string)  [unwired: 1 in]
              n181 = local read "igralec4"() -> (w777:string)
              n182 = Format Into String(w730) -> (resulting string=w731:string)  [unwired: 3 in, 1 out]
              n183 = local read "Povprecje4_tekma"() -> (w760:dbl)
              n184 = Concatenate Strings(w777, w762, "                          " ("string"), w731, "  cm" ("string"), "\r\n") -> (→"igralec4":string)
              n185 = Add(x="Lokalni Stevec 4", y=1.0) -> (x+y=w752:dbl)
              "Stevilo skokov tocka 4" <- w752
              n186 = local read "igralec4 2"() -> (w768:string)
              n187 = local write "Lokalni Stevec 4"(w752) -> ()
              n188 = xnode "Formula"("X1"=w760, "X2"=w733, "X3"=w730) -> ("Result"=→"Povprecje4_tekma":dbl)  [unwired: 1 in, 1 out]
              n189 = Number To Decimal String(number=w752) -> (decimal integer string=w751:string)  [unwired: 1 in]
              n190 = Concatenate Strings(w768, w751, w763, w731, w764, w765) -> (→"igralec4 2":string)
              n191 = local read "igralec4 3"() -> (w766:string)
              n192 = local read "Povprecje4_set"() -> (w759:dbl)
              n193 = local read "Povprecje4_tocka"() -> (w758:dbl)
              n194 = Subtract(x=w733, y="ID_prejsnji_set4") -> (x-y=w754:dbl)
              "Stevilo skokov set 4" <- w754
              n195 = Number To Decimal String(number=w754) -> (decimal integer string=w753:string)  [unwired: 1 in]
              n196 = Concatenate Strings(w766, w753, w763, w731, w764, w765) -> (→"igralec4 3":string)
              n197 = xnode "Formula"("X1"=w758, "X2"=w752, "X3"=w730) -> ("Result"=→"Povprecje4_tocka":dbl)  [unwired: 1 in, 1 out]
              n198 = xnode "Formula"("X1"=w759, "X2"=w754, "X3"=w730) -> ("Result"=→"Povprecje4_set":dbl)  [unwired: 1 in, 1 out]
              n199 = local read "Writing"() -> (w732:string[])
              n200 = global read "filePath.vi" "Path"() -> (w746:path)
              n201 = Tick Count (ms)() -> (millisecond timer value=w728:u32)
              n202 = global read "Stevci_Globals.vi" "zacetni cas"() -> (w722:dbl)
              n203 = Number To Decimal String(number=w733) -> (decimal integer string=w743:string)  [unwired: 1 in]
              n204 = Format Into String(w730) -> (resulting string=w729:string)  [unwired: 3 in, 1 out]
              n205 = Subtract(x=w728, y=w722) -> (x-y=w727:dbl)
              n206 = Concatenate Strings("Številka skoka: " ("string"), w743) -> (w740:string)
              n207 = Concatenate Strings(w729, " cm" ("string")) -> (w739:string)
              n208 = String To Path(string="skoki_igralec4.tdms") -> (path=w748:path)
              n209 = Replace Array Subset(array=w732, new element=w739, index=0) -> (w737:string[])
              n210 = Build Path(base path=w746, name or relative path=w748) -> (appended path=w749:path)
              n211 = local read "Time Stamp"() -> (w719:timestamp)
              n212 = global read "Stevci_Globals.vi" "casovna razlika"() -> (w721:dbl)
              n213 = Subtract(x=w727, y=w721) -> (x-y=w726:dbl)
              n214 = Divide(x=w726, y=1000.0) -> (x/y=w724:dbl)
              n215 = TDMS Open(10:T2."open or create" ("operation (0:open)"), 11:w749) -> (3:w750:refnum<k34>)  [unwired: 5 in, 1 out]
              n216 = Add(x=w724, y=w719) -> (x+y=w723:timestamp)
              n217 = Format Date/Time String(seconds (now)=w723) -> (date/time string=w720:string)  [unwired: 2 in]
              n218 = Replace Array Subset(array=w737, new element=w720, index=1) -> (w735:string[])
              n219 = TDMS Write(0:w750, 5:"Skoki" ("group name in (Untitled)"), 7:w740, 9:w735) -> (4:w734:refnum<k34>)  [unwired: 2 in, 3 out]
              n220 = TDMS Close(11:w734) -> ()  [unwired: 1 in, 2 out]
              "Stevilo skokov tekma 4" <- w733
            }
          }
        }
        n221 = global write "belezenje.vi" "ID"(0.0 ("ID")) -> ()
      }
      frame 5 {
        n222 = global read "Stevci_Globals.vi" "Števec skokov 5"() -> (w825:dbl)
        n223 = local read "Lokalni Stevec 5"() -> (w823:dbl)
        n224 = Subtract(x=w825, y=w823) -> (x-y=w824:dbl)
        n225 = for {
          N: w824 -> [_]
          tunnel: w823 -> [w830]
          i -> [w831]
          n226 = global read "Jumps_Globals.vi" "Jumps 5"() -> (w828:dbl[][])
          n227 = Add(x=w830, y=w831) -> (x+y=w827:dbl)
          n228 = Index Array(array=w828, index (row)=w827, index (col)=3 ("index")) -> (element=w833:dbl)
          n229 = Index Array(array=w828, index (row)=w827, index (col)=5 ("index")) -> (element=w826:dbl)
          n230 = case shown="1, Default" w833 {
            tunnel: w833 -> [_ w848]
            tunnel: w826 -> [_ w889]
            frame 0 {
            }
            frame 1, Default {
              w879 = "  cm" ("string")
              w878 = "                          " ("string")
              w880 = "\r\n"
              n231 = xnode "Formula"("X1"=w889) -> ("Result"=w845:dbl)  [unwired: 1 in, 1 out]
              n232 = Number To Decimal String(number=w848) -> (decimal integer string=w877:string)  [unwired: 1 in]
              n233 = local read "igralec5"() -> (w892:string)
              n234 = Format Into String(w845) -> (resulting string=w846:string)  [unwired: 3 in, 1 out]
              n235 = local read "Povprecje5_tekma"() -> (w875:dbl)
              n236 = Concatenate Strings(w892, w877, "                          " ("string"), w846, "  cm" ("string"), "\r\n") -> (→"igralec5":string)
              n237 = Add(x="Lokalni Stevec 5", y=1.0) -> (x+y=w867:dbl)
              "Stevilo skokov tocka 5" <- w867
              n238 = local read "igralec5 2"() -> (w883:string)
              n239 = local write "Lokalni Stevec 5"(w867) -> ()
              n240 = xnode "Formula"("X1"=w875, "X2"=w848, "X3"=w845) -> ("Result"=→"Povprecje5_tekma":dbl)  [unwired: 1 in, 1 out]
              n241 = Number To Decimal String(number=w867) -> (decimal integer string=w866:string)  [unwired: 1 in]
              n242 = Concatenate Strings(w883, w866, w878, w846, w879, w880) -> (→"igralec5 2":string)
              n243 = local read "igralec5 3"() -> (w881:string)
              n244 = local read "Povprecje5_set"() -> (w874:dbl)
              n245 = local read "Povprecje5_tocka"() -> (w873:dbl)
              n246 = Subtract(x=w848, y="ID_prejsnji_set5") -> (x-y=w869:dbl)
              "Stevilo skokov set 5" <- w869
              n247 = Number To Decimal String(number=w869) -> (decimal integer string=w868:string)  [unwired: 1 in]
              n248 = Concatenate Strings(w881, w868, w878, w846, w879, w880) -> (→"igralec5 3":string)
              n249 = xnode "Formula"("X1"=w873, "X2"=w867, "X3"=w845) -> ("Result"=→"Povprecje5_tocka":dbl)  [unwired: 1 in, 1 out]
              n250 = xnode "Formula"("X1"=w874, "X2"=w869, "X3"=w845) -> ("Result"=→"Povprecje5_set":dbl)  [unwired: 1 in, 1 out]
              n251 = global read "filePath.vi" "Path"() -> (w861:path)
              n252 = local read "Writing"() -> (w847:string[])
              n253 = Number To Decimal String(number=w848) -> (decimal integer string=w858:string)  [unwired: 1 in]
              n254 = Format Into String(w845) -> (resulting string=w844:string)  [unwired: 3 in, 1 out]
              n255 = global read "Stevci_Globals.vi" "zacetni cas"() -> (w836:dbl)
              n256 = Tick Count (ms)() -> (millisecond timer value=w843:u32)
              n257 = Concatenate Strings("Številka skoka: " ("string"), w858) -> (w855:string)
              n258 = Concatenate Strings(w844, " cm" ("string")) -> (w854:string)
              n259 = String To Path(string="skoki_igralec5.tdms") -> (path=w863:path)
              n260 = global read "Stevci_Globals.vi" "casovna razlika"() -> (w835:dbl)
              n261 = Replace Array Subset(array=w847, new element=w854, index=0) -> (w852:string[])
              n262 = Build Path(base path=w861, name or relative path=w863) -> (appended path=w864:path)
              n263 = Subtract(x=w843, y=w836) -> (x-y=w842:dbl)
              n264 = Subtract(x=w842, y=w835) -> (x-y=w841:dbl)
              n265 = TDMS Open(10:T2."open or create" ("operation (0:open)"), 11:w864) -> (3:w865:refnum<k34>)  [unwired: 5 in, 1 out]
              n266 = local read "Time Stamp"() -> (w834:timestamp)
              n267 = Divide(x=w841, y=1000.0) -> (x/y=w839:dbl)
              n268 = Add(x=w839, y=w834) -> (x+y=w838:timestamp)
              n269 = Format Date/Time String(seconds (now)=w838) -> (date/time string=w837:string)  [unwired: 2 in]
              n270 = Replace Array Subset(array=w852, new element=w837, index=1) -> (w850:string[])
              n271 = TDMS Write(0:w865, 5:"Skoki" ("group name in (Untitled)"), 7:w855, 9:w850) -> (4:w849:refnum<k34>)  [unwired: 2 in, 3 out]
              n272 = TDMS Close(11:w849) -> ()  [unwired: 1 in, 2 out]
              "Stevilo skokov tekma 5" <- w848
            }
          }
        }
        n273 = global write "belezenje.vi" "ID"(0.0 ("ID")) -> ()
      }
      frame 6 {
        n274 = global read "Stevci_Globals.vi" "Števec skokov 6"() -> (w940:dbl)
        n275 = local read "Lokalni Stevec 6"() -> (w938:dbl)
        n276 = Subtract(x=w940, y=w938) -> (x-y=w939:dbl)
        n277 = for {
          N: w939 -> [_]
          tunnel: w938 -> [w945]
          i -> [w946]
          n278 = global read "Jumps_Globals.vi" "Jumps 6"() -> (w941:dbl[][])
          n279 = Add(x=w945, y=w946) -> (x+y=w943:dbl)
          n280 = Index Array(array=w941, index (row)=w943, index (col)=3 ("index")) -> (element=w948:dbl)
          n281 = Index Array(array=w941, index (row)=w943, index (col)=5 ("index")) -> (element=w942:dbl)
          n282 = case shown="1, Default" w948 {
            tunnel: w948 -> [_ w972]
            tunnel: w942 -> [_ w1004]
            frame 0 {
            }
            frame 1, Default {
              w994 = "  cm" ("string")
              w993 = "                          " ("string")
              w995 = "\r\n"
              n283 = xnode "Formula"("X1"=w1004) -> ("Result"=w960:dbl)  [unwired: 1 in, 1 out]
              n284 = Number To Decimal String(number=w972) -> (decimal integer string=w992:string)  [unwired: 1 in]
              n285 = local read "igralec6"() -> (w1007:string)
              n286 = Format Into String(w960) -> (resulting string=w961:string)  [unwired: 3 in, 1 out]
              n287 = local read "Povprecje6_tekma"() -> (w990:dbl)
              n288 = Concatenate Strings(w1007, w992, "                          " ("string"), w961, "  cm" ("string"), "\r\n") -> (→"igralec6":string)
              n289 = Add(x="Lokalni Stevec 6", y=1.0) -> (x+y=w982:dbl)
              "Stevilo skokov tocka 6" <- w982
              n290 = local read "igralec6 2"() -> (w998:string)
              n291 = xnode "Formula"("X1"=w990, "X2"=w972, "X3"=w960) -> ("Result"=→"Povprecje6_tekma":dbl)  [unwired: 1 in, 1 out]
              n292 = local write "Lokalni Stevec 6"(w982) -> ()
              n293 = Number To Decimal String(number=w982) -> (decimal integer string=w981:string)  [unwired: 1 in]
              n294 = Concatenate Strings(w998, w981, w993, w961, w994, w995) -> (→"igralec6 2":string)
              n295 = local read "igralec6 3"() -> (w996:string)
              n296 = local read "Povprecje6_set"() -> (w989:dbl)
              n297 = local read "Povprecje6_tocka"() -> (w988:dbl)
              n298 = Subtract(x=w972, y="ID_prejsnji_set6") -> (x-y=w984:dbl)
              "Stevilo skokov set 6" <- w984
              n299 = Number To Decimal String(number=w984) -> (decimal integer string=w983:string)  [unwired: 1 in]
              n300 = Concatenate Strings(w996, w983, w993, w961, w994, w995) -> (→"igralec6 3":string)
              n301 = xnode "Formula"("X1"=w988, "X2"=w982, "X3"=w960) -> ("Result"=→"Povprecje6_tocka":dbl)  [unwired: 1 in, 1 out]
              n302 = xnode "Formula"("X1"=w989, "X2"=w984, "X3"=w960) -> ("Result"=→"Povprecje6_set":dbl)  [unwired: 1 in, 1 out]
              n303 = global read "Stevci_Globals.vi" "zacetni cas"() -> (w952:dbl)
              n304 = global read "filePath.vi" "Path"() -> (w976:path)
              n305 = Tick Count (ms)() -> (millisecond timer value=w958:u32)
              n306 = Number To Decimal String(number=w972) -> (decimal integer string=w971:string)  [unwired: 1 in]
              n307 = Format Into String(w960) -> (resulting string=w959:string)  [unwired: 3 in, 1 out]
              n308 = global read "Stevci_Globals.vi" "casovna razlika"() -> (w951:dbl)
              n309 = Subtract(x=w958, y=w952) -> (x-y=w957:dbl)
              n310 = Concatenate Strings("Številka skoka: " ("string"), w971) -> (w968:string)
              n311 = Concatenate Strings(w959, " cm" ("string")) -> (w967:string)
              n312 = String To Path(string="skoki_igralec6.tdms") -> (path=w978:path)
              n313 = Subtract(x=w957, y=w951) -> (x-y=w956:dbl)
              n314 = Replace Array Subset(array="Writing", new element=w967, index=0) -> (w965:string[])
              n315 = Build Path(base path=w976, name or relative path=w978) -> (appended path=w979:path)
              n316 = local read "Time Stamp"() -> (w949:timestamp)
              n317 = Divide(x=w956, y=1000.0) -> (x/y=w954:dbl)
              n318 = TDMS Open(10:T2."open or create" ("operation (0:open)"), 11:w979) -> (3:w980:refnum<k34>)  [unwired: 5 in, 1 out]
              n319 = Add(x=w954, y=w949) -> (x+y=w953:timestamp)
              n320 = Format Date/Time String(seconds (now)=w953) -> (date/time string=w950:string)  [unwired: 2 in]
              n321 = Replace Array Subset(array=w965, new element=w950, index=1) -> (w963:string[])
              n322 = TDMS Write(0:w980, 5:"Skoki" ("group name in (Untitled)"), 7:w968, 9:w963) -> (4:w962:refnum<k34>)  [unwired: 2 in, 3 out]
              n323 = TDMS Close(11:w962) -> ()  [unwired: 1 in, 2 out]
              "Stevilo skokov tekma 6" <- w972
            }
          }
        }
        n324 = global write "belezenje.vi" "ID"(0.0 ("ID")) -> ()
      }
    }
    n325 = global read "senzorji.vi" "3"() -> (→"Senzor 3":bool)
    n326 = case shown="True" "?" {
      frame False {
      }
      frame True {
        w353 = 0.0 ("Povprecje1_tocka")
        w354 = 0.0 ("Lokalni Stevec")
        w356 = 0.0 ("Numeric")
        n327 = Concatenate Strings("Številka skoka   Višina skoka ", "\r\n") -> (w355:string)
        n328 = global write "Stevci_Globals.vi" "Števec skokov 2"(w356) -> ()
        n329 = global write "Stevci_Globals.vi" "Števec skokov"(w356) -> ()
        n330 = global write "Stevci_Globals.vi" "Števec skokov 3"(w356) -> ()
        n331 = global write "Stevci_Globals.vi" "Števec skokov 4"(w356) -> ()
        n332 = global write "Stevci_Globals.vi" "Števec skokov 5"(w356) -> ()
        n333 = global write "Stevci_Globals.vi" "Števec skokov 6"(w356) -> ()
        n334 = local write "igralec5 2"(w355) -> ()
        n335 = local write "igralec6 2"(w355) -> ()
        n336 = local write "igralec4 2"(w355) -> ()
        n337 = local write "igralec1 2"(w355) -> ()
        n338 = local write "igralec3 2"(w355) -> ()
        n339 = local write "igralec2 2"(w355) -> ()
        n340 = Initialize Array(0.0 ("element"), 30 ("dimension size"), 6 ("dimension size")) -> (w357:dbl[][])
        n341 = global write "Jumps_Globals.vi" "Jumps"(w357) -> ()
        n342 = global write "Jumps_Globals.vi" "Jumps 6"(w357) -> ()
        n343 = global write "Jumps_Globals.vi" "Jumps 4"(w357) -> ()
        n344 = global write "Jumps_Globals.vi" "Jumps 5"(w357) -> ()
        n345 = global write "Jumps_Globals.vi" "Jumps 3"(w357) -> ()
        n346 = local write "Lokalni Stevec"(w354) -> ()
        n347 = local write "Lokalni Stevec 2"(w354) -> ()
        n348 = local write "Lokalni Stevec 4"(w354) -> ()
        n349 = local write "Povprecje4_tocka"(w353) -> ()
        n350 = local write "Lokalni Stevec 5"(w354) -> ()
        n351 = local write "Povprecje5_tocka"(w353) -> ()
        n352 = local write "Povprecje6_tocka"(w353) -> ()
        n353 = local write "Povprecje1_tocka"(w353) -> ()
        n354 = local write "Povprecje3_tocka"(w353) -> ()
        n355 = local write "Povprecje2_tocka"(w353) -> ()
        n356 = local write "Lokalni Stevec 6"(w354) -> ()
        n357 = local write "Lokalni Stevec 3"(w354) -> ()
        n358 = global write "Jumps_Globals.vi" "Jumps 2"(w357) -> ()
      }
    }
    n359 = global read "senzorji.vi" "5"() -> (→"Senzor 5":bool)
    n360 = global read "senzorji.vi" "6"() -> (→"Senzor 6":bool)
    n361 = global read "senzorji.vi" "4"() -> (→"Senzor 4":bool)
    n362 = global read "senzorji.vi" "bat 3"() -> (→"baterija 3":dbl)
    n363 = global read "senzorji.vi" "bat 1"() -> (→"baterija 1":dbl)
    n364 = global read "senzorji.vi" "bat 2"() -> (→"baterija 2":dbl)
    n365 = global read "senzorji.vi" "bat 6"() -> (→"baterija 6":dbl)
    n366 = global read "senzorji.vi" "bat 5"() -> (→"baterija 5":dbl)
    n367 = global read "senzorji.vi" "bat 4"() -> (→"baterija 4":dbl)
    n368 = global read "senzorji.vi" "Numeric"() -> (w94:dbl)
    n369 = global read "senzorji.vi" "Numeric 2"() -> (w89:dbl)
    n370 = Tick Count (ms)() -> (millisecond timer value=w93:u32)
    n371 = Tick Count (ms)() -> (millisecond timer value=w88:u32)
    n372 = Subtract(x=w93, y=w94) -> (x-y=w92:dbl)
    n373 = Subtract(x=w88, y=w89) -> (x-y=w87:dbl)
    n374 = Greater?(x=5000.0, y=w92) -> (0:w90:bool)
    n375 = Greater?(x=5000.0, y=w87) -> (0:w85:bool)
    n376 = global write "senzorji.vi" "1"(w90) -> ()
    n377 = global write "senzorji.vi" "2"(w85) -> ()
    n378 = global read "senzorji.vi" "Numeric 3"() -> (w84:dbl)
    n379 = global read "senzorji.vi" "Numeric 4"() -> (w79:dbl)
    n380 = Tick Count (ms)() -> (millisecond timer value=w83:u32)
    n381 = Tick Count (ms)() -> (millisecond timer value=w78:u32)
    n382 = case shown="True" "?" {
      frame False {
      }
      frame True {
        n383 = local read "String 2"() -> (w298:string)
        n384 = global read "filePath.vi" "Tdms_path"() -> (w238:path)
        n385 = local read "String"() -> (w315:string)
        n386 = global read "belezenje.vi" "zaporedni_set"() -> (w322:dbl)
        n387 = Number To Decimal String(number=w322) -> (decimal integer string=w237:string)  [unwired: 1 in]
        n388 = Concatenate Strings("Set ", w237) -> (w233:string)
        n389 = Concatenate Strings("\\" ("string"), w298) -> (w303:string)
        n390 = Concatenate Strings(w233, "\\skoki_igralec2.tdms") -> (w294:string)
        n391 = Concatenate Strings(w233, w303) -> (w302:string)
        n392 = Concatenate Strings("Set ", w237) -> (w312:string)
        n393 = Concatenate Strings("\\" ("string"), w315) -> (w313:string)
        n394 = String To Path(string=w294) -> (path=w295:path)
        n395 = Add(x=1.0, y=w322) -> (x+y=w344:dbl)
        n396 = Concatenate Strings(w302, ".tdms" ("string")) -> (w301:string)
        n397 = Concatenate Strings(w312, w313) -> (w311:string)
        n398 = Concatenate Strings(w312, "\\skoki_igralec1.tdms") -> (w317:string)
        n399 = Number To Decimal String(number=w344) -> (decimal integer string=w343:string)  [unwired: 1 in]
        n400 = String To Path(string=w301) -> (path=w299:path)
        n401 = local read "Povprecje2_set"() -> (w120:dbl)
        n402 = String To Path(string=w317) -> (path=w323:path)
        n403 = Concatenate Strings(w311, ".tdms" ("string")) -> (w310:string)
        n404 = global write "belezenje.vi" "zaporedni_set"(w344) -> ()
        n405 = local read "Writing"() -> (w196:string[])
        n406 = Concatenate Strings("Set ", w343) -> (w342:string)
        n407 = String To Path(string=w310) -> (path=w321:path)
        n408 = Build Path(base path=w238, name or relative path=w299) -> (appended path=w307:path)
        n409 = Build Path(base path=w238, name or relative path=w295) -> (appended path=w305:path)
        n410 = String To Path(string=w342) -> (path=w348:path)
        n411 = Build Path(base path=w238, name or relative path=w348) -> (appended path=w347:path)
        n412 = Build Path(base path=w238, name or relative path=w321) -> (appended path=w320:path)
        n413 = local read "Povprecje1_set"() -> (w122:dbl)
        n414 = Concatenate Strings("Številka skoka   Višina skoka ", "\r\n") -> (w350:string)
        n415 = Build Path(base path=w238, name or relative path=w323) -> (appended path=w308:path)
        n416 = local read "Writing"() -> (w224:string[])
        n417 = Create Folder(path (use dialog)=w347) -> (created path=w346:path)  [unwired: 2 in, 2 out]
        n418 = local write "igralec1 3"(w350) -> ()
        n419 = Copy(9:TRUE ("overwrite (F)"), 10:w307, 11:w305) -> (0:w198:errorcluster, 3:w199:path)  [unwired: 2 in, 1 out]
        n420 = local write "igralec3 3"(w350) -> ()
        n421 = local write "igralec4 3"(w350) -> ()
        n422 = local write "igralec2 3"(w350) -> ()
        n423 = local write "igralec6 3"(w350) -> ()
        n424 = local write "igralec5 3"(w350) -> ()
        n425 = Copy(9:TRUE ("overwrite (F)"), 10:w320, 11:w308) -> (0:w216:errorcluster, 3:w230:path)  [unwired: 2 in, 1 out]
        n426 = global write "filePath.vi" "Path"(w346) -> ()
        n427 = Less?(x=w120, y=0.0) -> (x < y?=w202:bool)
        n428 = TDMS Open(8:w198, 10:T2."open" ("operation (0:open)"), 11:w199) -> (0:w201:errorcluster, 3:w210:refnum<k34>)  [unwired: 4 in]
        n429 = Less?(x=w122, y=0.0) -> (x < y?=w218:bool)
        n430 = TDMS Open(8:w216, 10:T2."open" ("operation (0:open)"), 11:w230) -> (0:w215:errorcluster, 3:w227:refnum<k34>)  [unwired: 4 in]
        n431 = Boolean To (0,1)(Boolean=w202) -> (0, 1=w195:i16)
        n432 = Format Into String(w120) -> (resulting string=w119:string)  [unwired: 3 in, 1 out]
        n433 = Boolean To (0,1)(Boolean=w218) -> (0, 1=w217:i16)
        n434 = Format Into String(w122) -> (resulting string=w121:string)  [unwired: 3 in, 1 out]
        n435 = Concatenate Strings(w119, " cm" ("string")) -> (w206:string)
        n436 = Replace Array Subset(array=w196, new element=w206, index=0) -> (w205:string[])
        n437 = TDMS Write(0:w210, 5:"Skoki" ("group name in (Untitled)"), 7:"AVG" ("channel name(s) in (Untitled)"), 9:w205, 11:w201) -> (4:w209:refnum<k34>, 15:w200:errorcluster)  [unwired: 1 in, 2 out]
        n438 = Concatenate Strings(w121, " cm" ("string")) -> (w222:string)
        n439 = Replace Array Subset(array=w224, new element=w222, index=0) -> (w221:string[])
        n440 = TDMS Write(0:w227, 5:"Skoki" ("group name in (Untitled)"), 7:"AVG" ("channel name(s) in (Untitled)"), 9:w221, 11:w215) -> (4:w226:refnum<k34>, 15:w214:errorcluster)  [unwired: 1 in, 2 out]
        n441 = TDMS Close(8:w200, 11:w209) -> (0:→"error out 2":errorcluster)  [unwired: 1 out]
        n442 = TDMS Close(8:w214, 11:w226) -> (0:→"error out":errorcluster)  [unwired: 1 out]
        n443 = local write "Povprecje1_set"(w217) -> ()
        n444 = local write "Povprecje2_set"(w195) -> ()
        n445 = local read "String 3"() -> (w280:string)
        n446 = local read "String 4"() -> (w266:string)
        n447 = global read "Jump_Globals.vi" "Jump 6"() -> (w326:dbl[])
        n448 = global read "Jump_Globals.vi" "Jump 4"() -> (w332:dbl[])
        n449 = global read "Jump_Globals.vi" "Jump 5"() -> (w329:dbl[])
        n450 = global read "Jump_Globals.vi" "Jump 1"() -> (w341:dbl[])
        n451 = global read "Jump_Globals.vi" "Jump 3"() -> (w335:dbl[])
        n452 = global read "Jump_Globals.vi" "Jump 2"() -> (w338:dbl[])
        n453 = Concatenate Strings("Set ", w237) -> (w234:string)
        n454 = Concatenate Strings("Set ", w237) -> (w235:string)
        n455 = Index Array(array=w326, index=3) -> (element=w324:dbl)
        n456 = Index Array(array=w332, index=3) -> (element=w330:dbl)
        n457 = Concatenate Strings("\\" ("string"), w266) -> (w275:string)
        n458 = Concatenate Strings("\\" ("string"), w280) -> (w289:string)
        n459 = Index Array(array=w329, index=3) -> (element=w327:dbl)
        n460 = Index Array(array=w341, index=3) -> (element=w340:dbl)
        n461 = Index Array(array=w335, index=3) -> (element=w333:dbl)
        n462 = Index Array(array=w338, index=3) -> (element=w336:dbl)
        n463 = Concatenate Strings(w234, "\\skoki_igralec3.tdms") -> (w281:string)
        n464 = Concatenate Strings(w234, w289) -> (w288:string)
        n465 = Concatenate Strings(w235, "\\skoki_igralec4.tdms") -> (w267:string)
        n466 = local read "Povprecje4_set"() -> (w116:dbl)
        n467 = Concatenate Strings(w235, w275) -> (w274:string)
        n468 = local write "ID_prejsnji_set3"(w333) -> ()
        n469 = local write "ID_prejsnji_set1"(w340) -> ()
        n470 = String To Path(string=w281) -> (path=w282:path)
        n471 = local write "ID_prejsnji_set5"(w327) -> ()
        n472 = local write "ID_prejsnji_set6"(w324) -> ()
        n473 = local write "ID_prejsnji_set2"(w336) -> ()
        n474 = local write "ID_prejsnji_set4"(w330) -> ()
        n475 = Concatenate Strings(w288, ".tdms" ("string")) -> (w287:string)
        n476 = String To Path(string=w267) -> (path=w268:path)
        n477 = Concatenate Strings(w274, ".tdms" ("string")) -> (w273:string)
        n478 = String To Path(string=w287) -> (path=w285:path)
        n479 = String To Path(string=w273) -> (path=w271:path)
        n480 = local read "Povprecje3_set"() -> (w118:dbl)
        n481 = local read "Writing"() -> (w178:string[])
        n482 = Build Path(base path=w238, name or relative path=w268) -> (appended path=w277:path)
        n483 = local read "Writing"() -> (w160:string[])
        n484 = Build Path(base path=w238, name or relative path=w285) -> (appended path=w293:path)
        n485 = Build Path(base path=w238, name or relative path=w271) -> (appended path=w279:path)
        n486 = Build Path(base path=w238, name or relative path=w282) -> (appended path=w291:path)
        n487 = Less?(x=w116, y=0.0) -> (x < y?=w166:bool)
        n488 = Copy(9:TRUE ("overwrite (F)"), 10:w279, 11:w277) -> (0:w162:errorcluster, 3:w161:path)  [unwired: 2 in, 1 out]
        n489 = Boolean To (0,1)(Boolean=w166) -> (0, 1=w159:i16)
        n490 = Less?(x=w118, y=0.0) -> (x < y?=w184:bool)
        n491 = TDMS Open(8:w162, 10:T2."open" ("operation (0:open)"), 11:w161) -> (0:w165:errorcluster, 3:w174:refnum<k34>)  [unwired: 4 in]
        n492 = Copy(9:TRUE ("overwrite (F)"), 10:w293, 11:w291) -> (0:w179:errorcluster, 3:w180:path)  [unwired: 2 in, 1 out]
        n493 = Format Into String(w116) -> (resulting string=w115:string)  [unwired: 3 in, 1 out]
        n494 = Concatenate Strings(w115, " cm" ("string")) -> (w170:string)
        n495 = Boolean To (0,1)(Boolean=w184) -> (0, 1=w177:i16)
        n496 = Format Into String(w118) -> (resulting string=w117:string)  [unwired: 3 in, 1 out]
        n497 = Replace Array Subset(array=w160, new element=w170, index=0) -> (w169:string[])
        n498 = TDMS Open(8:w179, 10:T2."open" ("operation (0:open)"), 11:w180) -> (0:w183:errorcluster, 3:w192:refnum<k34>)  [unwired: 4 in]
        n499 = TDMS Write(0:w174, 5:"Skoki" ("group name in (Untitled)"), 7:"AVG" ("channel name(s) in (Untitled)"), 9:w169, 11:w165) -> (4:w173:refnum<k34>, 15:w164:errorcluster)  [unwired: 1 in, 2 out]
        n500 = Concatenate Strings(w117, " cm" ("string")) -> (w188:string)
        n501 = Replace Array Subset(array=w178, new element=w188, index=0) -> (w187:string[])
        n502 = local write "Povprecje3_set"(w177) -> ()
        n503 = TDMS Close(8:w164, 11:w173) -> (0:→"error out 3":errorcluster)  [unwired: 1 out]
        n504 = TDMS Write(0:w192, 5:"Skoki" ("group name in (Untitled)"), 7:"AVG" ("channel name(s) in (Untitled)"), 9:w187, 11:w183) -> (4:w191:refnum<k34>, 15:w182:errorcluster)  [unwired: 1 in, 2 out]
        n505 = local write "Povprecje4_set"(w159) -> ()
        n506 = TDMS Close(8:w182, 11:w191) -> (0:→"error out 4":errorcluster)  [unwired: 1 out]
        n507 = local read "String 5"() -> (w252:string)
        n508 = local read "String 6"() -> (w236:string)
        n509 = Concatenate Strings("Set ", w237) -> (w231:string)
        n510 = Concatenate Strings("Set ", w237) -> (w232:string)
        n511 = Concatenate Strings("\\" ("string"), w236) -> (w247:string)
        n512 = Concatenate Strings(w231, "\\skoki_igralec6.tdms") -> (w239:string)
        n513 = Concatenate Strings(w231, w247) -> (w246:string)
        n514 = Concatenate Strings("\\" ("string"), w252) -> (w261:string)
        n515 = Concatenate Strings(w232, "\\skoki_igralec5.tdms") -> (w253:string)
        n516 = String To Path(string=w239) -> (path=w240:path)
        n517 = Concatenate Strings(w232, w261) -> (w260:string)
        n518 = Concatenate Strings(w246, ".tdms" ("string")) -> (w245:string)
        n519 = String To Path(string=w253) -> (path=w254:path)
        n520 = String To Path(string=w245) -> (path=w243:path)
        n521 = Concatenate Strings(w260, ".tdms" ("string")) -> (w259:string)
        n522 = String To Path(string=w259) -> (path=w257:path)
        n523 = Build Path(base path=w238, name or relative path=w243) -> (appended path=w251:path)
        n524 = local read "Writing"() -> (w142:string[])
        n525 = local read "Writing"() -> (w124:string[])
        n526 = Build Path(base path=w238, name or relative path=w240) -> (appended path=w249:path)
        n527 = Build Path(base path=w238, name or relative path=w257) -> (appended path=w265:path)
        n528 = local read "Povprecje6_set"() -> (w112:dbl)
        n529 = Build Path(base path=w238, name or relative path=w254) -> (appended path=w263:path)
        n530 = Copy(9:TRUE ("overwrite (F)"), 10:w251, 11:w249) -> (0:w125:errorcluster, 3:w126:path)  [unwired: 2 in, 1 out]
        n531 = local read "Povprecje5_set"() -> (w114:dbl)
        n532 = Copy(9:TRUE ("overwrite (F)"), 10:w265, 11:w263) -> (0:w144:errorcluster, 3:w145:path)  [unwired: 2 in, 1 out]
        n533 = Less?(x=w114, y=0.0) -> (x < y?=w148:bool)
        n534 = Less?(x=w112, y=0.0) -> (x < y?=w130:bool)
        n535 = TDMS Open(8:w144, 10:T2."open" ("operation (0:open)"), 11:w145) -> (0:w147:errorcluster, 3:w156:refnum<k34>)  [unwired: 4 in]
        n536 = TDMS Open(8:w125, 10:T2."open" ("operation (0:open)"), 11:w126) -> (0:w129:errorcluster, 3:w138:refnum<k34>)  [unwired: 4 in]
        n537 = Boolean To (0,1)(Boolean=w148) -> (0, 1=w141:i16)
        n538 = Boolean To (0,1)(Boolean=w130) -> (0, 1=w123:i16)
        n539 = Format Into String(w114) -> (resulting string=w113:string)  [unwired: 3 in, 1 out]
        n540 = Format Into String(w112) -> (resulting string=w111:string)  [unwired: 3 in, 1 out]
        n541 = Concatenate Strings(w113, " cm" ("string")) -> (w152:string)
        n542 = Replace Array Subset(array=w142, new element=w152, index=0) -> (w151:string[])
        n543 = Concatenate Strings(w111, " cm" ("string")) -> (w134:string)
        n544 = Replace Array Subset(array=w124, new element=w134, index=0) -> (w133:string[])
        n545 = TDMS Write(0:w156, 5:"Skoki" ("group name in (Untitled)"), 7:"AVG" ("channel name(s) in (Untitled)"), 9:w151, 11:w147) -> (4:w155:refnum<k34>, 15:w146:errorcluster)  [unwired: 1 in, 2 out]
        n546 = TDMS Write(0:w138, 5:"Skoki" ("group name in (Untitled)"), 7:"AVG" ("channel name(s) in (Untitled)"), 9:w133, 11:w129) -> (4:w137:refnum<k34>, 15:w128:errorcluster)  [unwired: 1 in, 2 out]
        n547 = local write "Povprecje5_set"(w141) -> ()
        n548 = local write "Povprecje6_set"(w123) -> ()
        n549 = TDMS Close(8:w146, 11:w155) -> (0:→"error out 5":errorcluster)  [unwired: 1 out]
        n550 = TDMS Close(8:w128, 11:w137) -> (0:→"error out 6":errorcluster)  [unwired: 1 out]
      }
    }
    n551 = Subtract(x=w83, y=w84) -> (x-y=w82:dbl)
    n552 = Subtract(x=w78, y=w79) -> (x-y=w77:dbl)
    n553 = Greater?(x=5000.0, y=w82) -> (0:w80:bool)
    n554 = Greater?(x=5000.0, y=w77) -> (0:w75:bool)
    n555 = global write "senzorji.vi" "3"(w80) -> ()
    n556 = global write "senzorji.vi" "4"(w75) -> ()
    n557 = global read "senzorji.vi" "Numeric 5"() -> (w69:dbl)
    n558 = Tick Count (ms)() -> (millisecond timer value=w68:u32)
    n559 = global read "senzorji.vi" "Numeric 6"() -> (w74:dbl)
    n560 = Tick Count (ms)() -> (millisecond timer value=w73:u32)
    n561 = Subtract(x=w68, y=w69) -> (x-y=w67:dbl)
    n562 = Greater?(x=5000.0, y=w67) -> (0:w65:bool)
    n563 = Subtract(x=w73, y=w74) -> (x-y=w72:dbl)
    n564 = Greater?(x=5000.0, y=w72) -> (0:w70:bool)
    n565 = global write "senzorji.vi" "5"(w65) -> ()
    n566 = global write "senzorji.vi" "6"(w70) -> ()
    n567 = local read "String 6"() -> (w104:string)
    n568 = local read "String 5"() -> (w105:string)
    n569 = local read "String 4"() -> (w103:string)
    n570 = local read "String 3"() -> (w102:string)
    n571 = local read "String 2"() -> (w106:string)
    n572 = local read "String"() -> (w101:string)
    n573 = local write "String 18"(w106) -> ()
    n574 = local write "String 17"(w101) -> ()
    n575 = local write "String 16"(w106) -> ()
    n576 = local write "String 15"(w105) -> ()
    n577 = local write "String 14"(w103) -> ()
    n578 = local write "String 13"(w102) -> ()
    n579 = local write "String 12"(w104) -> ()
    n580 = local write "String 11"(w105) -> ()
    n581 = local write "String 10"(w104) -> ()
    n582 = local write "String 9"(w103) -> ()
    n583 = local write "String 8"(w102) -> ()
    n584 = local write "String 7"(w101) -> ()
  }
  n585 = Tick Count (ms)() -> (millisecond timer value=w4:u32)
  n586 = Build Path(base path=w26, name or relative path=path "Labview_posnetki" ("file path")) -> (appended path=w23:path)
  n587 = global write "Stevci_Globals.vi" "zacetni cas"(w4) -> ()
  n588 = global read "belezenje.vi" "zaporedni_set"() -> (w22:dbl)
  n589 = Build Path(base path=w23, name or relative path=w2) -> (appended path=w17:path)
  n590 = Get Date/Time In Seconds() -> (seconds since 1Jan1904=→"Time Stamp":timestamp)
  n591 = Initialize Array(0.0 ("element"), 30 ("dimension size"), 6 ("dimension size")) -> (w39:dbl[][])
  n592 = global write "filePath.vi" "Tdms_path"(w17) -> ()
  n593 = global write "Jumps_Globals.vi" "Jumps 3"(w39) -> ()
  n594 = global write "Jumps_Globals.vi" "Jumps 4"(w39) -> ()
  n595 = global write "Jumps_Globals.vi" "Jumps 2"(w39) -> ()
  n596 = global write "Jumps_Globals.vi" "Jumps 5"(w39) -> ()
  n597 = global write "Jumps_Globals.vi" "Jumps 6"(w39) -> ()
  n598 = global write "Jumps_Globals.vi" "Jumps"(w39) -> ()
  n599 = Number To Decimal String(number=w22) -> (decimal integer string=w20:string)  [unwired: 1 in]
  n600 = Concatenate Strings("Set ", w20) -> (w18:string)
  n601 = String To Path(string=w18) -> (path=w21:path)
  n602 = Build Path(base path=w17, name or relative path=w21) -> (appended path=w16:path)
  n603 = Create Folder(path (use dialog)=w16) -> ()  [unwired: 2 in, 3 out]
  n604 = global write "senzorji.vi" "6"(w3) -> ()
  n605 = global write "senzorji.vi" "3"(w3) -> ()
  n606 = global write "senzorji.vi" "1"(w3) -> ()
  n607 = global write "senzorji.vi" "2"(w3) -> ()
  n608 = global write "senzorji.vi" "4"(w3) -> ()
  n609 = global write "senzorji.vi" "5"(w3) -> ()
  n610 = global write "filePath.vi" "Path"(w16) -> ()
  n611 = global write "Stevci_Globals.vi" "Števec vseh skokov"(0.0 ("Števec skokov")) -> ()
  n612 = global write "Stevci_Globals.vi" "Števec skokov"(0.0 ("Števec skokov")) -> ()
  n613 = Open VI Reference(vi path=path "receiveUdp.vi") -> (vi reference=w56:refnum<vi>)  [unwired: 5 in, 1 out]
  n614 = global write "Stevci_Globals.vi" "Števec vseh skokov 2"(0.0 ("Števec skokov")) -> ()
  n615 = global write "Stevci_Globals.vi" "Števec skokov 2"(0.0 ("Števec skokov")) -> ()
  n616 = Concatenate Strings("Številka skoka   Višina skoka ", "\r\n") -> (w29:string)
  n617 = local write "igralec1"(w29) -> ()
  n618 = local write "igralec2 2"(w29) -> ()
  n619 = local write "igralec1 2"(w29) -> ()
  n620 = local write "igralec2"(w29) -> ()
  n621 = local write "igralec3 2"(w29) -> ()
  n622 = local write "igralec3"(w29) -> ()
  n623 = local write "igralec4 2"(w29) -> ()
  n624 = local write "igralec5 2"(w29) -> ()
  n625 = local write "igralec4"(w29) -> ()
  n626 = local write "igralec5"(w29) -> ()
  n627 = local write "igralec6"(w29) -> ()
  n628 = local write "igralec6 2"(w29) -> ()
  n629 = invoke class="VI" method="Run VI"(reference=w56, "Wait until done"=FALSE ("Wait Until Done")) -> (reference out=w55:refnum<vi>)  [unwired: 3 in, 4 out]
  n630 = local write "igralec4 3"(w29) -> ()
  n631 = local write "igralec2 3"(w29) -> ()
  n632 = local write "igralec3 3"(w29) -> ()
  n633 = local write "igralec5 3"(w29) -> ()
  n634 = local write "igralec6 3"(w29) -> ()
  n635 = local write "igralec1 3"(w29) -> ()
  n636 = global write "Stevci_Globals.vi" "Števec vseh skokov 3"(0.0 ("Števec skokov")) -> ()
  n637 = global write "Stevci_Globals.vi" "Števec skokov 3"(0.0 ("Števec skokov")) -> ()
  n638 = Close Reference(reference=w55) -> ()  [unwired: 1 in, 1 out]
  n639 = local write "String"("Vpiši igralca 1") -> ()
  n640 = local write "String 2"("Vpiši igralca 2") -> ()
  n641 = local write "String 3"("Vpiši igralca 3") -> ()
  n642 = local write "String 4"("Vpiši igralca 4") -> ()
  n643 = local write "String 6"("Vpiši igralca 6") -> ()
  n644 = local write "String 5"("Vpiši igralca 5") -> ()
  n645 = global write "belezenje.vi" "zaporedni_set"(1.0 ("zaporedni_set")) -> ()
  n646 = global write "Stevci_Globals.vi" "Števec vseh skokov 4"(0.0 ("Števec skokov")) -> ()
  n647 = local write "Povprecje1_tekma"(w9) -> ()
  n648 = local write "Povprecje1_tocka"(w9) -> ()
  n649 = local write "Povprecje1_set"(w9) -> ()
  n650 = local write "Povprecje2_tekma"(w9) -> ()
  n651 = local write "Povprecje2_tocka"(w9) -> ()
  n652 = global write "Stevci_Globals.vi" "Števec skokov 4"(0.0 ("Števec skokov")) -> ()
  n653 = local write "Povprecje2_set"(w9) -> ()
  n654 = Initialize Array("", 2 ("dimension size")) -> (w6:string[])
  n655 = local write "Writing"(w6) -> ()
  n656 = local write "Povprecje3_tekma"(w9) -> ()
  n657 = local write "Povprecje3_tocka"(w9) -> ()
  n658 = local write "Povprecje3_set"(w9) -> ()
  n659 = local write "Povprecje4_tocka"(w9) -> ()
  n660 = local write "Povprecje4_set"(w9) -> ()
  n661 = local write "Povprecje4_tekma"(w9) -> ()
  n662 = global write "Stevci_Globals.vi" "Števec vseh skokov 5"(0.0 ("Števec skokov")) -> ()
  n663 = global write "Stevci_Globals.vi" "Števec skokov 5"(0.0 ("Števec skokov")) -> ()
  n664 = local write "Povprecje5_tekma"(w9) -> ()
  n665 = local write "Povprecje5_tocka"(w9) -> ()
  n666 = local write "Povprecje5_set"(w9) -> ()
  n667 = local write "Povprecje6_tocka"(w9) -> ()
  n668 = local write "Povprecje6_set"(w9) -> ()
  n669 = local write "Povprecje6_tekma"(w9) -> ()
  n670 = global write "Stevci_Globals.vi" "Števec vseh skokov 6"(0.0 ("Števec skokov")) -> ()
  n671 = global write "Stevci_Globals.vi" "Števec skokov 6"(0.0 ("Števec skokov")) -> ()
  n672 = local write "ID_prejsnji_set1"(w8) -> ()
  n673 = local write "ID_prejsnji_set5"(w8) -> ()
  n674 = local write "ID_prejsnji_set4"(w8) -> ()
  n675 = local write "ID_prejsnji_set2"(w8) -> ()
  n676 = local write "ID_prejsnji_set3"(w8) -> ()
  n677 = local write "ID_prejsnji_set6"(w8) -> ()
